vi "Parse Uplink.vi"(8 "error in (no error)":errorcluster, 10 "Uplink":u8[][](array[numeric]) format="%02x") -> (0 "error out":errorcluster, 1 "Data":string, 2 "Response Code":string, 3 "Response Token":string, 4 "tChecksum Valid":bool, 5 "CP_DATA":u8[](array[numeric]), 6 "bChecksum Valid":bool)   [LabVIEW 2020]
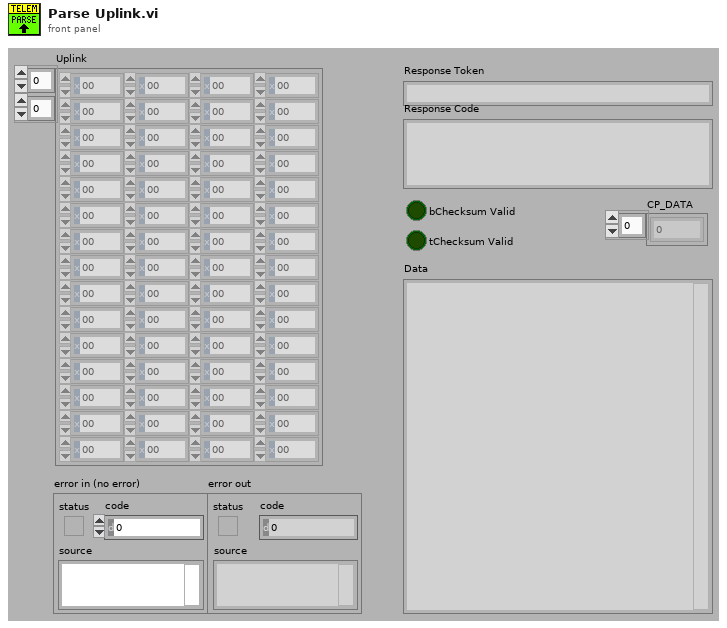
[diagram p1: front panel]
types:
  T1 = cluster{"FirstBlockFlag":u8, "respToken":u8, "cmdToken":u16, "cmdData":u8[], "b1ChkSum":u8, "tChkSum":u8, "tChkSumCalc":u8, "b1ChkSumCalc":u8}
  T2 = cluster{"Boolean array[0]":bool, "Boolean array[1]":bool, "Boolean array[2]":bool, "Boolean array[3]":bool, "Boolean array[4]":bool, "Boolean array[5]":bool, "Boolean array[6]":bool, "Boolean array[7]":bool}
  T3 = cluster{"Boolean array[0]":bool, "Boolean array[1]":bool, "Boolean array[2]":bool, "Boolean array[3]":bool, "Boolean array[4]":bool, "Boolean array[5]":bool, "Boolean array[6]":bool, "Boolean array[7]":bool, "Boolean array[8]":bool, "Boolean array[9]":bool, "Boolean array[10]":bool, "Boolean array[11]":bool, "Boolean array[12]":bool, "Boolean array[13]":bool, "Boolean array[14]":bool, "Boolean array[15]":bool}
  T4 = cluster{"DATA[0]":u8, "DATA[1]":u8, "DATA[2]":u8, "DATA[3]":u8, "DATA[4]":u8, "DATA[5]":u8, "DATA[6]":u8, "DATA[7]":u8}
  T5 = cluster{"[0]":string, "[1]":string, "[2]":string, "[3]":string, "[4]":string, "[5]":string, "[6]":string, "[7]":string, "[8]":string, "[9]":string}
  T6 = cluster{"DATA[0]":u8, "DATA[1]":u8, "DATA[2]":u8, "DATA[3]":u8, "DATA[4]":u8, "DATA[5]":u8, "DATA[6]":u8, "DATA[7]":u8, "DATA[8]":u8, "DATA[9]":u8, "DATA[10]":u8, "DATA[11]":u8, "DATA[12]":u8, "DATA[13]":u8, "DATA[14]":u8, "DATA[15]":u8}
  T7 = cluster{"[0]":u8, "[1]":u8, "[2]":u8, "[3]":u8, "[4]":u8, "[5]":u8, "[6]":u8, "[7]":u8, "[8]":u8, "[9]":u8, "[10]":u8, "[11]":u8, "[12]":u8, "[13]":u8, "[14]":u8, "[15]":u8, "[16]":u8, "[17]":u8, "[18]":u8, "[19]":u8, "[20]":u8, "[21]":u8, "[22]":u8, "[23]":u8, "[24]":u8, "[25]":u8, "[26]":u8, "[27]":u8, "[28]":u8, "[29]":u8, "[30]":u8, "[31]":u8, "[32]":u8, "[33]":u8, "[34]":u8, "[35]":u8, "[36]":u8, "[37]":u8, "[38]":u8, "[39]":u8, "[40]":u8, "[41]":u8, "[42]":u8, "[43]":u8, "[44]":u8, "[45]":u8, "[46]":u8, "[47]":u8, "[48]":u8, "[49]":u8, "[50]":u8, "[51]":u8, "[52]":u8, "[53]":u8}
  T8 = cluster{"DATA[0]":u8, "DATA[1]":u8, "DATA[2]":u8, "DATA[3]":u8, "DATA[4]":u8, "DATA[5]":u8, "DATA[6]":u8, "DATA[7]":u8, "DATA[8]":u8, "DATA[9]":u8, "DATA[10]":u8, "DATA[11]":u8, "DATA[12]":u8, "DATA[13]":u8, "DATA[14]":u8, "DATA[15]":u8, "DATA[16]":u8, "DATA[17]":u8, "DATA[18]":u8, "DATA[19]":u8, "DATA[20]":u8, "DATA[21]":u8, "DATA[22]":u8, "DATA[23]":u8, "DATA[24]":u8, "DATA[25]":u8, "DATA[26]":u8, "DATA[27]":u8, "DATA[28]":u8, "DATA[29]":u8, "DATA[30]":u8, "DATA[31]":u8, "DATA[32]":u8, "DATA[33]":u8, "DATA[34]":u8, "DATA[35]":u8, "DATA[36]":u8, "DATA[37]":u8, "DATA[38]":u8, "DATA[39]":u8, "DATA[40]":u8, "DATA[41]":u8, "DATA[42]":u8, "DATA[43]":u8, "DATA[44]":u8, "DATA[45]":u8, "DATA[46]":u8}
  T9 = cluster{"DATA[0]":u8, "DATA[1]":u8, "DATA[2]":u8, "DATA[3]":u8, "DATA[4]":u8, "DATA[5]":u8, "DATA[6]":u8, "DATA[7]":u8, "DATA[8]":u8, "DATA[9]":u8, "DATA[10]":u8, "DATA[11]":u8, "DATA[12]":u8, "DATA[13]":u8, "DATA[14]":u8, "DATA[15]":u8, "DATA[16]":u8, "DATA[17]":u8, "DATA[18]":u8, "DATA[19]":u8, "DATA[20]":u8, "DATA[21]":u8, "DATA[22]":u8, "DATA[23]":u8}
  T10 = cluster{"Boolean array[0]":bool, "Boolean array[1]":bool, "Boolean array[2]":bool, "Boolean array[3]":bool, "Boolean array[4]":bool, "Boolean array[5]":bool, "Boolean array[6]":bool, "Boolean array[7]":bool, "Boolean array[8]":bool}
  T11 = cluster{"[0]":u8, "[1]":u8, "[2]":u8, "[3]":u8, "[4]":u8, "[5]":u8, "[6]":u8, "[7]":u8, "[8]":u8, "[9]":u8}
  T12 = cluster{"DATA[0]":u8, "DATA[1]":u8, "DATA[2]":u8, "DATA[3]":u8, "DATA[4]":u8, "DATA[5]":u8, "DATA[6]":u8, "DATA[7]":u8, "DATA[8]":u8}
  T13 = cluster{"[0]":u8, "[1]":u8, "[2]":u8, "[3]":u8, "[4]":u8, "[5]":u8, "[6]":u8, "[7]":u8, "[8]":u8, "[9]":u8, "[10]":u8, "[11]":u8, "[12]":u8, "[13]":u8, "[14]":u8, "[15]":u8, "[16]":u8, "[17]":u8, "[18]":u8, "[19]":u8, "[20]":u8, "[21]":u8, "[22]":u8, "[23]":u8, "[24]":u8, "[25]":u8, "[26]":u8, "[27]":u8, "[28]":u8, "[29]":u8, "[30]":u8, "[31]":u8, "[32]":u8, "[33]":u8, "[34]":u8, "[35]":u8, "[36]":u8, "[37]":u8}
  T14 = cluster{"[0]":u8, "[1]":u8, "[2]":u8, "[3]":u8, "[4]":u8, "[5]":u8}
  T15 = cluster{"DATA[0]":u8, "DATA[1]":u8, "DATA[2]":u8, "DATA[3]":u8, "DATA[4]":u8, "DATA[5]":u8}
  T16 = cluster{"DATA[0]":u8, "DATA[1]":u8, "DATA[2]":u8, "DATA[3]":u8, "DATA[4]":u8, "DATA[5]":u8, "DATA[6]":u8, "DATA[7]":u8, "DATA[8]":u8, "DATA[9]":u8, "DATA[10]":u8, "DATA[11]":u8, "DATA[12]":u8, "DATA[13]":u8, "DATA[14]":u8, "DATA[15]":u8, "DATA[16]":u8}
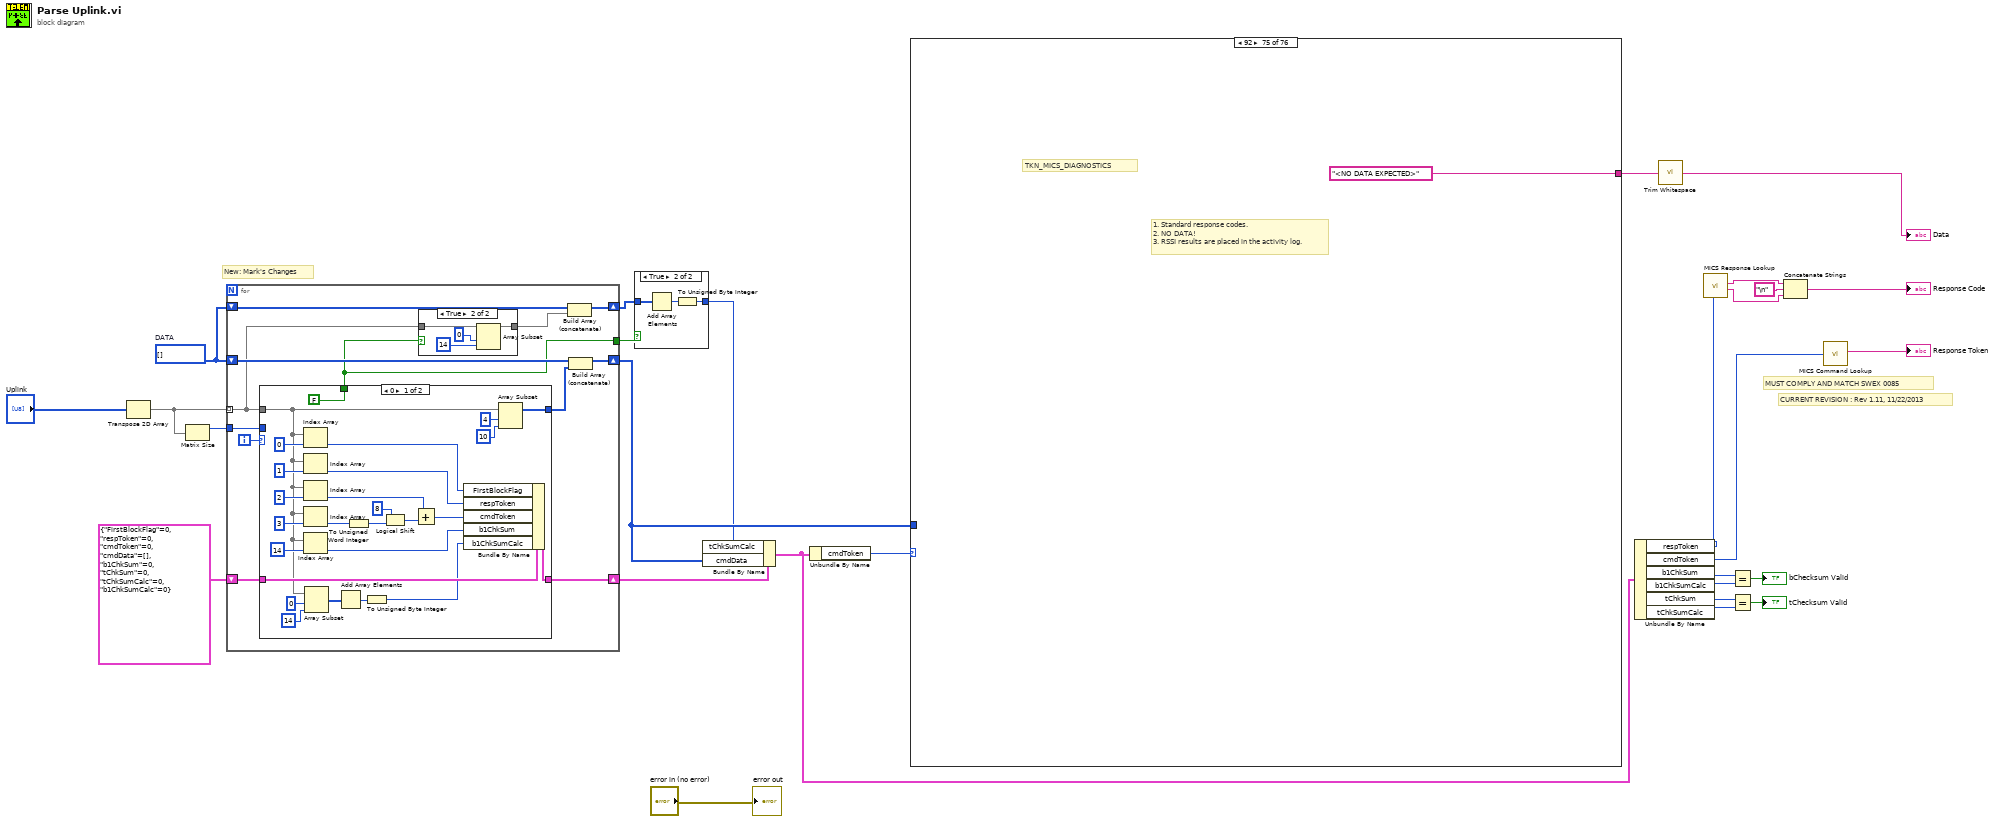
[diagram p0: block diagram]
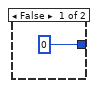
[diagram p2: hidden frame]
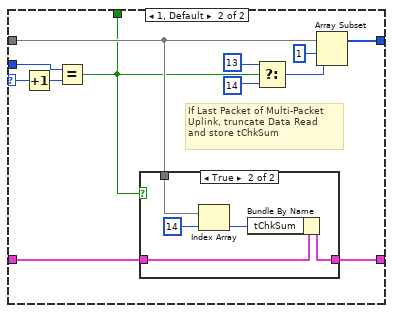
[diagram p4: hidden frame]
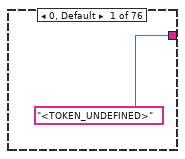
[diagram p6: hidden frame]
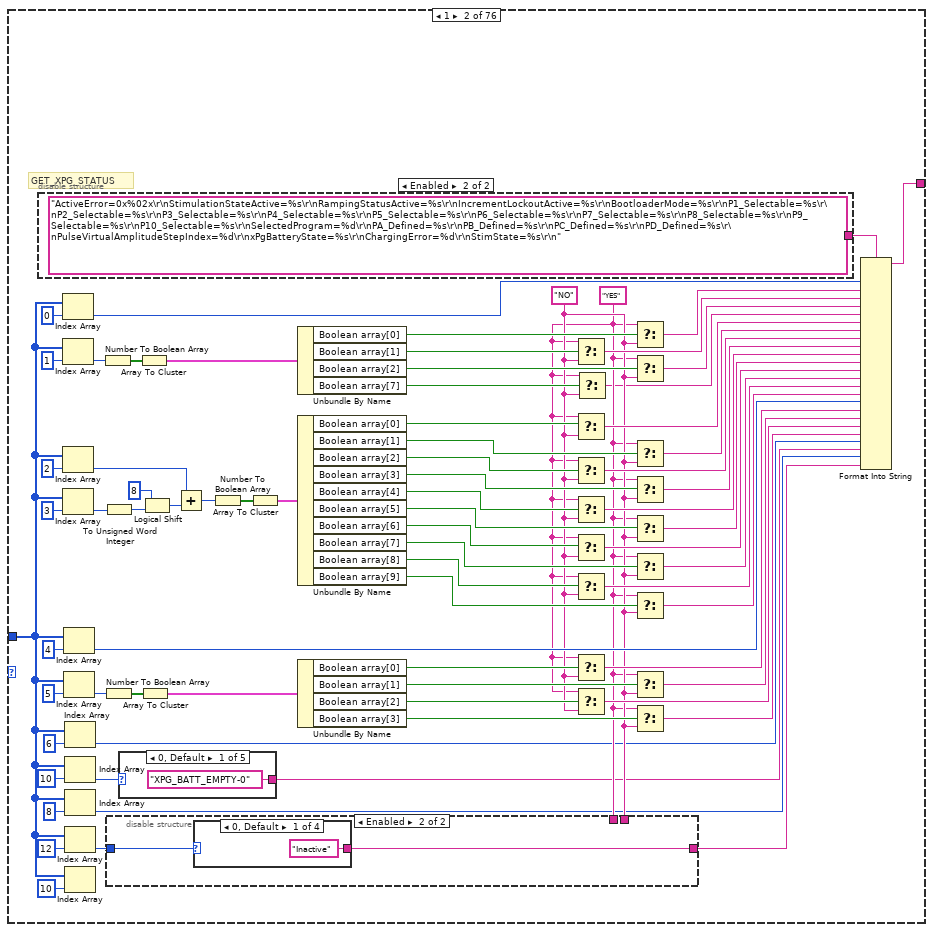
[diagram p7: hidden frame]
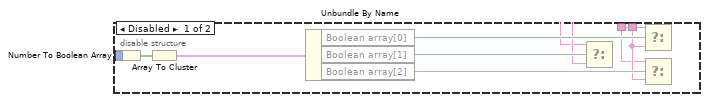
[diagram p8: hidden frame]
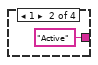
[diagram p9: hidden frame]
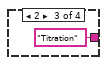
[diagram p10: hidden frame]
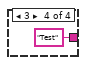
[diagram p11: hidden frame]
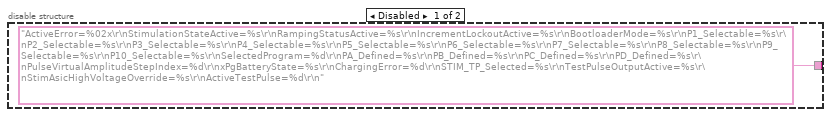
[diagram p12: hidden frame]
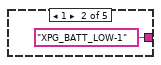
[diagram p13: hidden frame]
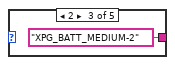
[diagram p14: hidden frame]
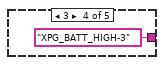
[diagram p15: hidden frame]
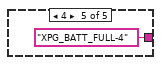
[diagram p16: hidden frame]
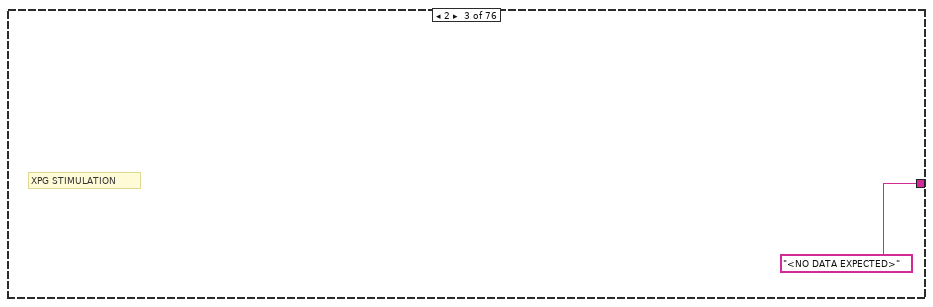
[diagram p17: hidden frame]
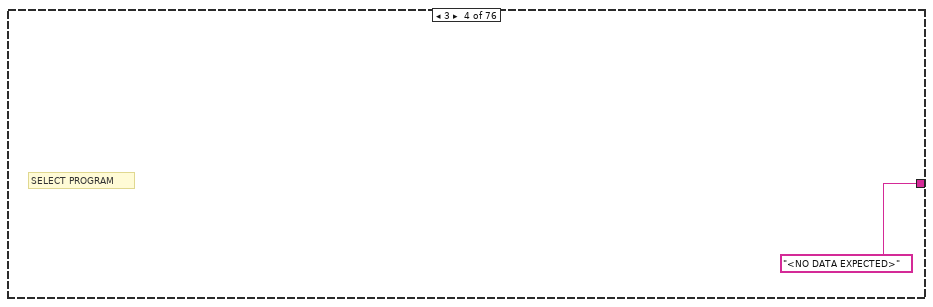
[diagram p18: hidden frame]
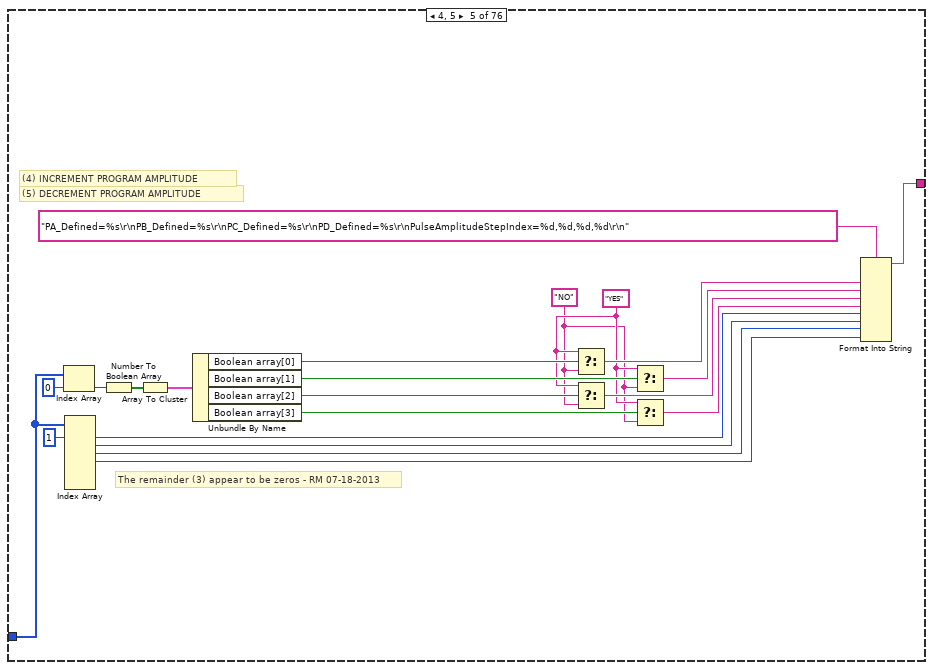
[diagram p19: hidden frame]
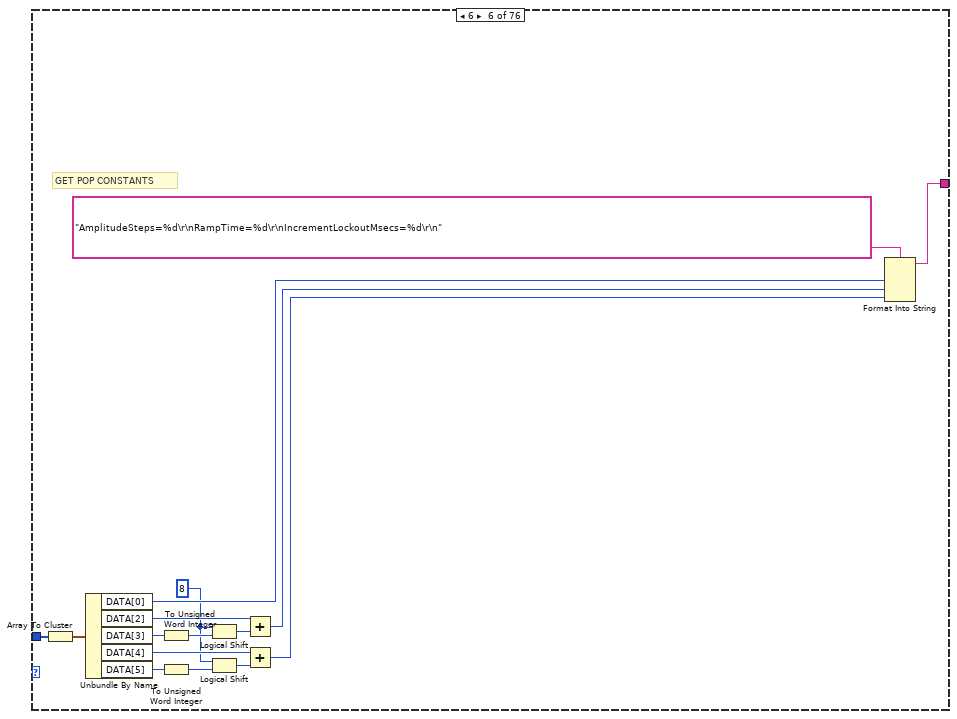
[diagram p20: hidden frame]
diagram:
  w12 = u8[] []  # DATA
  # "CURRENT REVISION : Rev 1.11, 11/22/2013"
  # "MUST COMPLY AND MATCH SWEX 0085"
  # "New: Mark's Changes"
  n1 = Transpose 2D Array(2D array="Uplink") -> (transposed array=w11:u8[][])
  n2 = Matrix Size(0:w11) -> (1:w9:i32)  [unwired: 1 out]
  n3 = for {
    tunnel: w11 -> [w31] mode=indexing
    shift-right: [w35] -> w28
    shift-left: w12 -> [w36]
    shift-right: [w38] -> w10
    shift-left: T1 {"FirstBlockFlag"=0, "respToken"=0, "cmdToken"=0, "cmdData"=[], "b1ChkSum"=0, "tChkSum"=0, "tChkSumCalc"=0, "b1ChkSumCalc"=0} -> [w39]
    tunnel: w9 -> [w37]
    shift-right: [w32] -> w13
    shift-left: w12 -> [w33]
    tunnel: [w29] -> w14
    i -> [w40]
    n4 = case shown="0" w40 {
      selector: w40 -> [_ w83]
      tunnel: w31 -> [w49 w73]
      tunnel: [w69 w79] -> w34
      tunnel: w39 -> [w63 w74]
      tunnel: [w62 w75] -> w38
      tunnel: w37 -> [_ w81]
      tunnel: [FALSE w72] -> w29
      frame 0 {
        n5 = Index Array(array=w49, index=0) -> (element=w61:u8)
        n6 = Index Array(array=w49, index=1) -> (element=w58:u8)
        n7 = Index Array(array=w49, index=2) -> (element=w53:u8)
        n8 = Index Array(array=w49, index=3) -> (element=w57:u8)
        n9 = Index Array(array=w49, index=14) -> (element=w60:u8)
        n10 = Array Subset(array=w49, index=0, length=14) -> (w46:u8[])
        n11 = Add Array Elements(numeric array=w46) -> (sum=w48:u8)
        n12 = To Unsigned Word Integer(number=w57) -> (unsigned 16bit integer=w59:u16)
        n13 = To Unsigned Byte Integer(number=w48) -> (unsigned 8bit integer=w47:u8)
        n14 = Logical Shift(y=i8 8, x=w59) -> (x << y=w55:u16)
        n15 = Add(x=w53, y=w55) -> (x+y=w54:u16)
        n16 = Bundle By Name(cluster=w63, "FirstBlockFlag"=w61, "respToken"=w58, "cmdToken"=w54, "b1ChkSum"=w60, "b1ChkSumCalc"=w47) -> (w62:T1)
        n17 = Array Subset(array=w49, index=4, length=10) -> (w69:u8[])
      }
      frame 1, Default {
        # "If Last Packet of Multi-Packet\nUplink, truncate Data Read\nand store tChkSum"
        n18 = Increment(x=w83) -> (x+1=w82:i32)
        n19 = Equal?(x=w81, y=w82) -> (x = y?=w72:bool)
        n20 = case shown="True" w72 {
          tunnel: [w84 w88] -> w75
          tunnel: w74 -> [w84 w89]
          tunnel: w73 -> [_ w86]
          frame False {
          }
          frame True {
            n21 = Index Array(array=w86, index=14) -> (element=w87:u8)
            n22 = Bundle By Name(cluster=w89, "tChkSum"=w87) -> (w88:T1)
          }
        }
        n23 = Select(t=13 ("length"), s=w72, f=14 ("length")) -> (s? t:f=w78:i32)
        n24 = Array Subset(array=w73, index=1, length=w78) -> (w79:u8[])
      }
    }
    n25 = case shown="True" w29 {
      tunnel: w31 -> [w41 w44]
      tunnel: [w41 w43] -> w30
      frame False {
      }
      frame True {
        n26 = Array Subset(array=w44, index=0, length=14) -> (w43:u8[])
      }
    }
    n27 = Build Array (concatenate)(w33, w30) -> (w32:u8[])
    n28 = Build Array (concatenate)(w36, w34) -> (w35:u8[])
  }
  n29 = case shown="True" w14 {
    tunnel: w13 -> [_ w91]
    tunnel: [u16 0 ("CRC16r") w92] -> w15
    frame False {
    }
    frame True {
      n30 = Add Array Elements(numeric array=w91) -> (sum=w93:u8)
      n31 = To Unsigned Byte Integer(number=w93) -> (unsigned 8bit integer=w92:u8)
    }
  }
  n32 = Bundle By Name(cluster=w10, "tChkSumCalc"=w15, "cmdData"=w28) -> (w19:T1)
  n33 = Unbundle By Name(w19) -> ("cmdToken"=w16:u16)
  n34 = case shown="92" w16 {
    tunnel: w28 -> [_ w104 _ _ w203 w221 w230 w312 w358 w363 w368 w384 _ w403 w408 w413 _ w419 w424 _ w439 w465 _ _ w473 _ w610 _ w635 _ w785 _ w794 _ w852 _ w899 _ w925 _ _ w954 w988 w1010 _ w1018 _ w1028 w1033 w1054 _ w1144 _ w1192 _ w1197 _ w1257 _ w1313 _ w1318 _ _ _ w1336 _ _ _ _ w1353 _ w1409 w1417 _ _]
    tunnel: ["<TOKEN_UNDEFINED>" w166 "<NO DATA EXPECTED>" "<NO DATA EXPECTED>" w213 w228 w289 w345 w359 w364 w369 w398 "<NO DATA EXPECTED>" w404 w409 w414 "<NO DATA EXPECTED>" w420 w425 "<NO DATA EXPECTED>" w440 w452 "<NO DATA EXPECTED>" "<NO DATA EXPECTED>" w512 "<NO DATA EXPECTED>" w613 "<NO DATA EXPECTED>" w700 "<NO DATA EXPECTED>" w789 "<NO DATA EXPECTED>" w799 "<NO DATA EXPECTED>" w857 "<NO DATA EXPECTED>" w902 "<NO DATA EXPECTED>" w928 "<NO DATA EXPECTED>" "<NO DATA EXPECTED>" ("format string") w955 w990 w1012 "<NO DATA EXPECTED>" w1022 "<NO DATA EXPECTED>" w1030 w1037 w1085 "<NO DATA EXPECTED>" w1145 "<NO DATA EXPECTED>" w1193 "<NO DATA EXPECTED>" w1205 "<NO DATA EXPECTED>" w1264 "<NO DATA EXPECTED>" w1314 "<NO DATA EXPECTED>" w1326 _ _ "<NO DATA EXPECTED>" w1344 _ _ _ _ w1354 "<NO DATA EXPECTED>" w1411 w1423 "<NO DATA EXPECTED>" "<TOKEN_UNDEFINED (0x7FAA)>"] -> w27
    frame 0, Default {
    }
    frame 1 {
      w102 = "NO"
      w101 = "YES"
      # "GET_XPG_STATUS"
      n35 = disable-structure shown="Enabled" {
        disable-tunnel: ["ActiveError=%02x\r\nStimulationStateActive=%s\r\nRampingStatusActive=%s\r\nIncrementLockoutActive=%s\r\nBootloaderMode=%s\r\nP1_Selectable=%s\r\nP2_Selectable=%s\r\nP3_Selectable=%s\r\nP4_Selectable=%s\r\nP5_Selectable=%s\r\nP6_Selectable=%s\r\nP7_Selectable=%s\r\nP8_Selectable=%s\r\nP9_Selectable=%s\r\nP10_Selectable=%s\r\nSelectedProgram=%d\r\nPA_Defined=%s\r\nPB_Defined=%s\r\nPC_Defined=%s\r\nPD_Defined=%s\r\nPulseVirtualAmplitudeStepIndex=%d\r\nxPgBatteryState=%s\r\nChargingError=%d\r\nSTIM_TP_Selected=%s\r\nTestPulseOutputActive=%s\r\nStimAsicHighVoltageOverride=%s\r\nActiveTestPulse=%d\r\n" ("format string") "ActiveError=0x%02x\r\nStimulationStateActive=%s\r\nRampingStatusActive=%s\r\nIncrementLockoutActive=%s\r\nBootloaderMode=%s\r\nP1_Selectable=%s\r\nP2_Selectable=%s\r\nP3_Selectable=%s\r\nP4_Selectable=%s\r\nP5_Selectable=%s\r\nP6_Selectable=%s\r\nP7_Selectable=%s\r\nP8_Selectable=%s\r\nP9_Selectable=%s\r\nP10_Selectable=%s\r\nSelectedProgram=%d\r\nPA_Defined=%s\r\nPB_Defined=%s\r\nPC_Defined=%s\r\nPD_Defined=%s\r\nPulseVirtualAmplitudeStepIndex=%d\r\nxPgBatteryState=%s\r\nChargingError=%d\r\nStimState=%s\r\n" ("format string")] -> w95
        frame Disabled {
        }
        frame Enabled {
        }
      }
      n36 = Index Array(array=w104, index=0) -> (element=w167:u8)
      n37 = Index Array(array=w104, index=1) -> (element=w151:u8)
      n38 = Index Array(array=w104, index=2) -> (element=w139:u8)
      n39 = Index Array(array=w104, index=3) -> (element=w140:u8)
      n40 = Index Array(array=w104, index=4) -> (element=w124:u8)
      n41 = Index Array(array=w104, index=5) -> (element=w122:u8)
      n42 = Index Array(array=w104, index=6) -> (element=w99:u8)
      n43 = Index Array(array=w104, index=10) -> (element=w109:u8)
      n44 = Index Array(array=w104, index=8) -> (element=w97:u8)
      n45 = Index Array(array=w104, index=12) -> (element=w106:u8)
      n46 = Index Array(array=w104, index=10) -> ()  [unwired: 1 out]
      n47 = Number To Boolean Array(number=w151) -> (Boolean array=w150:bool[])
      n48 = To Unsigned Word Integer(number=w140) -> (unsigned 16bit integer=w143:u16)
      n49 = Number To Boolean Array(number=w122) -> (Boolean array=w121:bool[])
      n50 = disable-structure shown="Enabled" {
        disable-tunnel: w106 -> [w176 w178]
        disable-tunnel: w102 -> [w170 _]
        disable-tunnel: w101 -> [w169 _]
        disable-tunnel: [_ w177] -> w96
        frame Disabled {
          n51 = Number To Boolean Array(number=w176) -> (Boolean array=w175:bool[])
          n52 = Array To Cluster(array=w175) -> (cluster=w174:T2)
          n53 = Unbundle By Name(w174) -> ("Boolean array[0]"=w173:bool, "Boolean array[1]"=w172:bool, "Boolean array[2]"=w171:bool)
          n54 = Select(t=w169, s=w172, f=w170) -> ()  [unwired: 1 out]
          n55 = Select(t=w169, s=w173, f=w170) -> ()  [unwired: 1 out]
          n56 = Select(t=w169, s=w171, f=w170) -> ()  [unwired: 1 out]
        }
        frame Enabled {
          n57 = case shown="0, Default" w178 {
            tunnel: ["Inactive" "Active" "Titration" "Test"] -> w177
            frame 0, Default {
            }
            frame 1 {
            }
            frame 2 {
            }
            frame 3 {
            }
          }
        }
      }
      n58 = case shown="0, Default" w109 {
        tunnel: ["XPG_BATT_EMPTY-0" "XPG_BATT_LOW-1" "XPG_BATT_MEDIUM-2" "XPG_BATT_HIGH-3" "XPG_BATT_FULL-4"] -> w98
        frame 0, Default {
        }
        frame 1 {
        }
        frame 2 {
        }
        frame 3 {
        }
        frame 4 {
        }
      }
      n59 = Array To Cluster(array=w150) -> (cluster=w149:T2)
      n60 = Array To Cluster(array=w121) -> (cluster=w120:T2)
      n61 = Logical Shift(y=i8 8, x=w143) -> (x << y=w141:u16)
      n62 = Add(x=w139, y=w141) -> (x+y=w137:u16)
      n63 = Number To Boolean Array(number=w137) -> (Boolean array=w138:bool[])
      n64 = Array To Cluster(array=w138) -> (cluster=w136:T3)
      n65 = Unbundle By Name(w149) -> ("Boolean array[0]"=w148:bool, "Boolean array[1]"=w147:bool, "Boolean array[2]"=w146:bool, "Boolean array[7]"=w103:bool)
      n66 = Unbundle By Name(w136) -> ("Boolean array[0]"=w135:bool, "Boolean array[1]"=w134:bool, "Boolean array[2]"=w133:bool, "Boolean array[3]"=w132:bool, "Boolean array[4]"=w131:bool, "Boolean array[5]"=w130:bool, "Boolean array[6]"=w129:bool, "Boolean array[7]"=w128:bool, "Boolean array[8]"=w127:bool, "Boolean array[9]"=w126:bool)
      n67 = Unbundle By Name(w120) -> ("Boolean array[0]"=w119:bool, "Boolean array[1]"=w118:bool, "Boolean array[2]"=w117:bool, "Boolean array[3]"=w116:bool)
      n68 = Select(t=w101, s=w147, f=w102) -> (s? t:f=w164:string)
      n69 = Select(t=w101, s=w135, f=w102) -> (s? t:f=w162:string)
      n70 = Select(t=w101, s=w133, f=w102) -> (s? t:f=w160:string)
      n71 = Select(t=w101, s=w131, f=w102) -> (s? t:f=w158:string)
      n72 = Select(t=w101, s=w129, f=w102) -> (s? t:f=w156:string)
      n73 = Select(t=w101, s=w127, f=w102) -> (s? t:f=w154:string)
      n74 = Select(t=w101, s=w119, f=w102) -> (s? t:f=w115:string)
      n75 = Select(t=w101, s=w117, f=w102) -> (s? t:f=w113:string)
      n76 = Select(t=w101, s=w103, f=w102) -> (s? t:f=w100:string)
      n77 = Select(t=w101, s=w148, f=w102) -> (s? t:f=w165:string)
      n78 = Select(t=w101, s=w146, f=w102) -> (s? t:f=w163:string)
      n79 = Select(t=w101, s=w134, f=w102) -> (s? t:f=w161:string)
      n80 = Select(t=w101, s=w132, f=w102) -> (s? t:f=w159:string)
      n81 = Select(t=w101, s=w130, f=w102) -> (s? t:f=w157:string)
      n82 = Select(t=w101, s=w128, f=w102) -> (s? t:f=w155:string)
      n83 = Select(t=w101, s=w126, f=w102) -> (s? t:f=w153:string)
      n84 = Select(t=w101, s=w118, f=w102) -> (s? t:f=w114:string)
      n85 = Select(t=w101, s=w116, f=w102) -> (s? t:f=w112:string)
      n86 = Format Into String(format string=w95, w167, w165, w164, w163, w100, w162, w161, w160, w159, w158, w157, w156, w155, w154, w153, w124, w115, w114, w113, w112, w99, w98, w97, w96) -> (resulting string=w166:string)  [unwired: 2 in, 1 out]
    }
    frame 2 {
      # "XPG STIMULATION"
    }
    frame 3 {
      # "SELECT PROGRAM"
    }
    frame 4, 5 {
      w196 = "NO"
      w197 = "YES"
      # "(5) DECREMENT PROGRAM AMPLITUDE"
      # "(4) INCREMENT PROGRAM AMPLITUDE"
      # "The remainder (3) appear to be zeros - RM 07-18-2013"
      n87 = Index Array(array=w203, index=0) -> (element=w211:u8)
      n88 = Index Array(array=w203, index #1=1 ("index")) -> (element #1=w198:u8, element #2=w194:u8, element #3=w193:u8, element #4=w192:u8)  [unwired: 6 in, 3 out]
      n89 = Number To Boolean Array(number=w211) -> (Boolean array=w210:bool[])
      n90 = Array To Cluster(array=w210) -> (cluster=w209:T2)
      n91 = Unbundle By Name(w209) -> ("Boolean array[0]"=w208:bool, "Boolean array[1]"=w207:bool, "Boolean array[2]"=w206:bool, "Boolean array[3]"=w205:bool)
      n92 = Select(t=w197, s=w208, f=w196) -> (s? t:f=w202:string)
      n93 = Select(t=w197, s=w206, f=w196) -> (s? t:f=w200:string)
      n94 = Select(t=w197, s=w207, f=w196) -> (s? t:f=w201:string)
      n95 = Select(t=w197, s=w205, f=w196) -> (s? t:f=w199:string)
      n96 = Format Into String(format string="PA_Defined=%s\r\nPB_Defined=%s\r\nPC_Defined=%s\r\nPD_Defined=%s\r\nPulseAmplitudeStepIndex=%d,%d,%d,%d\r\n", w202, w201, w200, w199, w198, w194, w193, w192) -> (resulting string=w213:string)  [unwired: 2 in, 1 out]
    }
    frame 6 {
      w214 = i8 8 ("y")
      # "GET POP CONSTANTS"
      n97 = Array To Cluster(array=w221) -> (cluster=w220:T4)
      n98 = Unbundle By Name(w220) -> ("DATA[0]"=w219:u8, "DATA[2]"=w218:u8, "DATA[3]"=w217:u8, "DATA[4]"=w216:u8, "DATA[5]"=w215:u8)
      n99 = To Unsigned Word Integer(number=w217) -> (unsigned 16bit integer=w227:u16)
      n100 = To Unsigned Word Integer(number=w215) -> (unsigned 16bit integer=w225:u16)
      n101 = Logical Shift(y=w214, x=w227) -> (x << y=w226:u16)
      n102 = Logical Shift(y=w214, x=w225) -> (x << y=w224:u16)
      n103 = Add(x=w218, y=w226) -> (x+y=w223:u16)
      n104 = Add(x=w216, y=w224) -> (x+y=w222:u16)
      n105 = Format Into String(format string="AmplitudeSteps=%d\r\nRampTime=%d\r\nIncrementLockoutMsecs=%d\r\n", w219, w223, w222) -> (resulting string=w228:string)  [unwired: 2 in, 1 out]
    }
    frame 7 {
      w232 = "NO"
      w270 = "YES"
      # "Convert MS DateTime\nto LV DateTime"
      # "GET PPC CONSTANTS"
      n106 = Array Subset(array=w230, index=0, length=30) -> (w286:u8[])
      n107 = Index Array(array=w230, index=30) -> (element=w278:u8)
      n108 = Index Array(array=w230, index=31) -> (element=w279:u8)
      n109 = Index Array(array=w230, index=32) -> (element=w275:u8)
      n110 = Index Array(array=w230, index=33) -> (element=w273:u8)
      n111 = Index Array(array=w230, index=34) -> (element=w257:u8)
      n112 = Index Array(array=w230, index=35) -> (element=w258:u8)
      n113 = Index Array(array=w230, index=36) -> (element=w249:u8)
      n114 = Index Array(array=w230, index=37) -> (element=w250:u8)
      n115 = Array Subset(array=w230, index=38, length=8) -> (w245:u8[])
      n116 = Index Array(array=w230, index=46) -> (element=w235:u8)
      n117 = Number To Boolean Array(number=w273) -> (Boolean array=w272:bool[])
      n118 = To Unsigned Word Integer(number=w279) -> (unsigned 16bit integer=w282:u16)
      n119 = To Unsigned Word Integer(number=w258) -> (unsigned 16bit integer=w261:u16)
      n120 = To Unsigned Word Integer(number=w250) -> (unsigned 16bit integer=w253:u16)
      n121 = Byte Array To String(unsigned byte array=w286) -> (string=w285:string)
      n122 = Array To Cluster(array=w272) -> (cluster=w271:T2)
      n123 = Logical Shift(y=i8 8, x=w282) -> (x << y=w280:u16)
      n124 = Logical Shift(y=i8 8, x=w261) -> (x << y=w259:u16)
      n125 = Logical Shift(y=i8 8, x=w253) -> (x << y=w251:u16)
      n126 = for {
        tunnel: w245 -> [w298] mode=indexing
        shift-right: [w292] -> w240
        shift-left: u64 0 ("y") -> [w293]
        tunnel: i8 8 ("y") -> [w296]
        i -> [w297]
        n127 = To Unsigned Quad Integer(1:w298) -> (0:w291:u64)
        n128 = Multiply(x=w296, y=w297) -> (x*y=w295:i32)
        n129 = Logical Shift(y=w295, x=w291) -> (x << y=w294:u64)
        n130 = Add(x=w293, y=w294) -> (x+y=w292:u64)
      }
      n131 = Add(x=w278, y=w280) -> (x+y=w277:u16)
      n132 = Unbundle By Name(w271) -> ("Boolean array[0]"=w268:bool, "Boolean array[1]"=w269:bool, "Boolean array[2]"=w267:bool)
      n133 = Add(x=w257, y=w259) -> (x+y=w256:u16)
      n134 = Add(x=w249, y=w251) -> (x+y=w248:u16)
      n135 = Select(t=w270, s=w268, f=w232) -> (s? t:f=w266:string)
      n136 = Select(t=w270, s=w267, f=w232) -> (s? t:f=w264:string)
      n137 = Multiply(x=u64 1904 ("y"), y=u64 31556926) -> (x*y=w238:u64)
      n138 = Quotient & Remainder(x=w240, y=u64 10000000) -> (floor(x/y)=w231:u64)  [unwired: 1 out]
      n139 = Select(t=w270, s=w269, f=w232) -> (s? t:f=w265:string)
      n140 = Subtract(x=w231, y=w238) -> (x-y=w234:u64)
      n141 = Format Date/Time String(seconds (now)=w234, UTC format=FALSE) -> (date/time string=w233:string)  [unwired: 1 in]
      n142 = Format Into String(format string="PPCText=%s\r\nPulseWidthStep=%d\r\nAmplitudeSteps=%d\r\nAllowIndividualPulseAmplitudeModification=%s\r\nAllowIndividualPulseWidthModification=%s\r\nAllowProgramFrequencyModification=%s\r\nRampTime=%d\r\nIncrementalLockoutMsecs=%d\r\nImplantDateTime=%s\r\nReplacementIntervalMonths=%d\r\n", w285, w277, w275, w266, w265, w264, w256, w248, w233, w235) -> (resulting string=w289:string)  [unwired: 2 in, 1 out]
    }
    frame 8 {
      w324 = "NO"
      w323 = "YES"
      # "GET_PROGRAM_NAMES"
      n143 = Index Array(array=w312, index=0) -> (element=w338:u8)
      n144 = Index Array(array=w312, index=1) -> (element=w339:u8)
      n145 = To Unsigned Word Integer(number=w339) -> (unsigned 16bit integer=w342:u16)
      n146 = Logical Shift(y=i8 8, x=w342) -> (x << y=w340:u16)
      n147 = Add(x=w338, y=w340) -> (x+y=w336:u16)
      n148 = for {
        N: 10 -> [_]
        tunnel: w312 -> [w355]
        tunnel: [w347] -> w311 mode=indexing
        i -> [w353]
        n149 = Multiply(x=16, y=w353) -> (x*y=w351:i32)
        n150 = Add(x=2, y=w351) -> (x+y=w349:i32)
        n151 = Array Subset(array=w355, index=w349, length=10) -> (w348:u8[])
        n152 = Byte Array To String(unsigned byte array=w348) -> (string=w347:string)
      }
      n153 = Number To Boolean Array(number=w336) -> (Boolean array=w337:bool[])
      n154 = Array To Cluster(array=w337) -> (cluster=w335:T3)
      n155 = Unbundle By Name(w335) -> ("Boolean array[0]"=w334:bool, "Boolean array[1]"=w333:bool, "Boolean array[2]"=w332:bool, "Boolean array[3]"=w331:bool, "Boolean array[4]"=w330:bool, "Boolean array[5]"=w329:bool, "Boolean array[6]"=w328:bool, "Boolean array[7]"=w327:bool, "Boolean array[8]"=w326:bool, "Boolean array[9]"=w325:bool)
      n156 = Array To Cluster(array=w311) -> (cluster=w310:T5)
      n157 = Unbundle(w310) -> ("[0]"=w308:string, "[1]"=w307:string, "[2]"=w306:string, "[3]"=w305:string, "[4]"=w304:string, "[5]"=w303:string, "[6]"=w302:string, "[7]"=w301:string, "[8]"=w300:string, "[9]"=w299:string)
      n158 = Select(t=w323, s=w334, f=w324) -> (s? t:f=w322:string)
      n159 = Select(t=w323, s=w332, f=w324) -> (s? t:f=w320:string)
      n160 = Select(t=w323, s=w330, f=w324) -> (s? t:f=w318:string)
      n161 = Select(t=w323, s=w328, f=w324) -> (s? t:f=w316:string)
      n162 = Select(t=w323, s=w326, f=w324) -> (s? t:f=w314:string)
      n163 = Select(t=w323, s=w333, f=w324) -> (s? t:f=w321:string)
      n164 = Select(t=w323, s=w331, f=w324) -> (s? t:f=w319:string)
      n165 = Select(t=w323, s=w329, f=w324) -> (s? t:f=w317:string)
      n166 = Select(t=w323, s=w327, f=w324) -> (s? t:f=w315:string)
      n167 = Select(t=w323, s=w325, f=w324) -> (s? t:f=w313:string)
      n168 = Format Into String(format string="P1_Selectable=%s\r\nP2_Selectable=%s\r\nP3_Selectable=%s\r\nP4_Selectable=%s\r\nP5_Selectable=%s\r\nP6_Selectable=%s\r\nP7_Selectable=%s\r\nP8_Selectable=%s\r\nP9_Selectable=%s\r\nP10_Selectable=%s\r\nP1_Name=%s\r\nP2_Name=%s\r\nP3_Name=%s\r\nP4_Name=%s\r\nP5_Name=%s\r\nP6_Name=%s\r\nP7_Name=%s\r\nP8_Name=%s\r\nP9_Name=%s\r\nP10_Name=%s\r\n", w322, w321, w320, w319, w318, w317, w316, w315, w314, w313, w308, w307, w306, w305, w304, w303, w302, w301, w300, w299) -> (resulting string=w345:string)  [unwired: 2 in, 1 out]
    }
    frame 9 {
      # "SET_PULSE_AMPLITUDE"
      n169 = Array To Cluster(array=w358) -> (cluster=w357:T4)
      n170 = Unbundle By Name(w357) -> ("DATA[0]"=w356:u8)
      n171 = Format Into String(format string="PulseAmplitudeStepIndex=%d\r\n", w356) -> (resulting string=w359:string)  [unwired: 2 in, 1 out]
    }
    frame 10 {
      # "INCREMENT_PULSE_AMPLITUDE"
      n172 = Array To Cluster(array=w363) -> (cluster=w362:T4)
      n173 = Unbundle By Name(w362) -> ("DATA[0]"=w361:u8)
      n174 = Format Into String(format string="PulseVirtualAmplitudeStepIndex=%d\r\n", w361) -> (resulting string=w364:string)  [unwired: 2 in, 1 out]
    }
    frame 11 {
      # "DECREMENT_PULSE_AMPLITUDE"
      n175 = Array To Cluster(array=w368) -> (cluster=w367:T4)
      n176 = Unbundle By Name(w367) -> ("DATA[0]"=w366:u8)
      n177 = Format Into String(format string="PulseVirtualAmplitudeStepIndex=%d\r\n", w366) -> (resulting string=w369:string)  [unwired: 2 in, 1 out]
    }
    frame 12 {
      w386 = "NO"
      w387 = "YES"
      # "GET_PULSE_WIDTHS"
      n178 = Array To Cluster(array=w384) -> (cluster=w385:T6)
      n179 = Unbundle By Name(w385) -> ("DATA[0]"=w383:u8, "DATA[3]"=w372:u8, "DATA[2]"=w371:u8, "DATA[5]"=w374:u8, "DATA[4]"=w373:u8, "DATA[7]"=w376:u8, "DATA[6]"=w375:u8, "DATA[9]"=w378:u8, "DATA[8]"=w377:u8)
      n180 = Join Numbers(hi=w372, lo=w371) -> ((hi.lo)=w382:u16)
      n181 = Join Numbers(hi=w374, lo=w373) -> ((hi.lo)=w381:u16)
      n182 = Join Numbers(hi=w376, lo=w375) -> ((hi.lo)=w380:u16)
      n183 = Join Numbers(hi=w378, lo=w377) -> ((hi.lo)=w379:u16)
      n184 = Number To Boolean Array(number=w383) -> (Boolean array=w397:bool[])
      n185 = Array To Cluster(array=w397) -> (cluster=w396:T2)
      n186 = Unbundle By Name(w396) -> ("Boolean array[0]"=w395:bool, "Boolean array[1]"=w394:bool, "Boolean array[2]"=w393:bool, "Boolean array[3]"=w392:bool)
      n187 = Select(t=w387, s=w395, f=w386) -> (s? t:f=w391:string)
      n188 = Select(t=w387, s=w393, f=w386) -> (s? t:f=w389:string)
      n189 = Select(t=w387, s=w394, f=w386) -> (s? t:f=w390:string)
      n190 = Select(t=w387, s=w392, f=w386) -> (s? t:f=w388:string)
      n191 = Format Into String(format string="PA_Defined=%s\r\nPB_Defined=%s\r\nPC_Defined=%s\r\nPD_Defined=%s\r\nPA_PulseWidth=%d\r\nPB_PulseWidth=%d\r\nPC_PulseWidth=%d\r\nPD_PulseWidth=%d\r\n", w391, w390, w389, w388, w382, w381, w380, w379) -> (resulting string=w398:string)  [unwired: 2 in, 1 out]
    }
    frame 13 {
      # "SET_PULSE_WIDTHS"
    }
    frame 14 {
      # "INCREMENT_PULSE_WIDTH"
      n192 = Array To Cluster(array=w403) -> (cluster=w402:T4)
      n193 = Unbundle By Name(w402) -> ("DATA[0]"=w401:u8)
      n194 = Format Into String(format string="PulseWidth=%d\r\n", w401) -> (resulting string=w404:string)  [unwired: 2 in, 1 out]
    }
    frame 15 {
      # "DECREMENT_PULSE_WIDTH"
      n195 = Array To Cluster(array=w408) -> (cluster=w407:T4)
      n196 = Unbundle By Name(w407) -> ("DATA[0]"=w406:u8)
      n197 = Format Into String(format string="PulseWidth=%d\r\n", w406) -> (resulting string=w409:string)  [unwired: 2 in, 1 out]
    }
    frame 16 {
      # "GET_PROGRAM_FREQUENCY"
      n198 = Array To Cluster(array=w413) -> (cluster=w412:T4)
      n199 = Unbundle By Name(w412) -> ("DATA[0]"=w411:u8)
      n200 = Format Into String(format string="ProgramFrequencyIndex=%d\r\n", w411) -> (resulting string=w414:string)  [unwired: 2 in, 1 out]
    }
    frame 17 {
      # "SET_PROGRAM_FREQUENCY"
    }
    frame 18 {
      # "INCREMENT_PROGRAM_FREQUENCY"
      n201 = Array To Cluster(array=w419) -> (cluster=w418:T4)
      n202 = Unbundle By Name(w418) -> ("DATA[0]"=w417:u8)
      n203 = Format Into String(format string="ProgramFrequencyIndex=%d\r\n", w417) -> (resulting string=w420:string)  [unwired: 2 in, 1 out]
    }
    frame 19 {
      # "DECREMENT_PROGRAM_FREQUENCY"
      n204 = Array To Cluster(array=w424) -> (cluster=w423:T4)
      n205 = Unbundle By Name(w423) -> ("DATA[0]"=w422:u8)
      n206 = Format Into String(format string="ProgramFrequencyIndex=%d\r\n", w422) -> (resulting string=w425:string)  [unwired: 2 in, 1 out]
    }
    frame 20 {
      # "INJECT_EVENT"
    }
    frame 21 {
      # "CHARGING_CONTROL"
      n207 = Array To Cluster(array=w439) -> (cluster=w438:T4)
      n208 = Unbundle By Name(w438) -> ("DATA[0]"=w433:u8, "DATA[1]"=w429:u8)
      n209 = And(x=240, y=w433) -> (x .and. y?=w435:i32)
      n210 = And(x=128, y=w433) -> (x .and. y?=w428:i32)
      n211 = And(x=w433, y=u8 15) -> (x .and. y?=w430:u8)
      n212 = case shown="48" w435 {
        tunnel: ["CHARGE_OFF-0" "CHARGE_PRE_CONDITION-1" "CHARGE_CONSTANT_CURRENT_FAST-2" "CHARGE_CONSTANT_CURRENT_SLOW-3" "CHARGE_COMPLETE-4" "CHARGE_ERROR-5" "CHARGE_CONSTANT_VOLTAGE_FAST-6" "CHARGE_CONSTANT_VOLTAGE_FAST-7"] -> w431
        frame 0, Default {
        }
        frame 16 {
        }
        frame 32 {
        }
        frame 48 {
        }
        frame 64 {
        }
        frame 80 {
        }
        frame 96 {
        }
        frame 112 {
        }
      }
      n213 = case shown="128" w428 {
        tunnel: ["NO" "YES"] -> w432
        frame 0, Default {
        }
        frame 128 {
          # "Charge Warning Bit Depricated"
        }
      }
      n214 = Format Into String(format string="ChargingState=%s\r\nChargeWarning=%s\r\nTemperatureLevel=%d\r\nIPG_ReceivedLevel=%d\r\n", w431, w432, w430, w429) -> (resulting string=w440:string)  [unwired: 2 in, 1 out]
    }
    frame 22 {
      # "GET_XPG_IDENTITY"
      n215 = Array Subset(array=w465, index=0, length=10) -> (w466:u8[])
      n216 = Array Subset(array=w465, index=10 ("length"), length=20) -> (w467:u8[])
      n217 = Array Subset(array=w465, index=30 ("length"), length=10) -> (w468:u8[])
      n218 = Byte Array To String(unsigned byte array=w466) -> (string=w458:string)
      n219 = Byte Array To String(unsigned byte array=w467) -> (string=w457:string)
      n220 = Byte Array To String(unsigned byte array=w468) -> (string=w456:string)
      n221 = Format Into String(format string="ModelNumber=%s\r\nSerialNumber=%s\r\nFirmwareVersion=%s\r\n", w458, w457, w456) -> (resulting string=w453:string)  [unwired: 2 in, 1 out]
      n222 = Search and Replace String(replace all?=TRUE ("replace all? (F)"), input string=w453, search string="\u0000") -> (result string=w452:string)  [unwired: 5 in, 3 out]
    }
    frame 23 {
      # "SET_XPG_IDENTITY"
    }
    frame 24 {
      # "RESTORE_PROGRAM_DEFAULTS"
    }
    frame 25 {
      w487 = "NO"
      w486 = "YES"
      # "GET_PROGRAM_DEFINITION"
      n223 = Index Array(array=w473, index=0) -> (element=w474:u8)
      n224 = Index Array(array=w473, index=2) -> (element=w508:u8)
      n225 = Index Array(array=w473, index=3) -> (element=w506:u8)
      n226 = Index Array(array=w473, index=28) -> (element=w478:u8)
      n227 = Index Array(array=w473, index=29) -> (element=w484:u8)
      n228 = for {
        N: 4 -> [_]
        tunnel: w473 -> [w565]
        shift-right: [w559] -> w477
        shift-left: "" -> [w560]
        i -> [w514]
        w524 = 8 ("index")
        w564 = 54 ("length")
        n229 = Multiply(x=w514, y=w564) -> (x*y=w562:i32)
        n230 = Add(x=30 ("index"), y=w562) -> (x+y=w563:i32)
        n231 = Array Subset(array=w565, index=w563, length=w564) -> (w521:u8[])
        n232 = case shown="3" w514 {
          tunnel: ["\r\n-- PULSE PA --\r\nPulseNamePA=%s\r\nAmplitudeLowLimitPA=%d\r\nAmplitudeStepPA=%d\r\nAmplitudeStepIndexPA=%d\r\nPulseWidthLowLimitPA=%d\r\nPulseWidthHighLimitPA=%d\r\nPulseWidthPA=%d\r\n%s" ("format string") "\r\n-- PULSE PB --\r\nPulseNamePB=%s\r\nAmplitudeLowLimitPB=%d\r\nAmplitudeStepPB=%d\r\nAmplitudeStepIndexPB=%d\r\nPulseWidthLowLimitPB=%d\r\nPulseWidthHighLimitPB=%d\r\nPulseWidthPB=%d\r\n%s" ("format string") "\r\n-- PULSE PC --\r\nPulseNamePC=%s\r\nAmplitudeLowLimitPC=%d\r\nAmplitudeStepPC=%d\r\nAmplitudeStepIndexPC=%d\r\nPulseWidthLowLimitPC=%d\r\nPulseWidthHighLimitPC=%d\r\nPulseWidthPC=%d\r\n%s" ("format string") "\r\n-- PULSE PD --\r\nPulseNamePD=%s\r\nAmplitudeLowLimitPD=%d\r\nAmplitudeStepPD=%d\r\nAmplitudeStepIndexPD=%d\r\nPulseWidthLowLimitPD=%d\r\nPulseWidthHighLimitPD=%d\r\nPulseWidthPD=%d\r\n%s" ("format string")] -> w556
          frame 0, Default {
          }
          frame 1 {
          }
          frame 2 {
          }
          frame 3 {
          }
        }
        n233 = Array Subset(array=w521, index=28, length=26) -> (w518:u8[])
        n234 = Array To Cluster(array=w521) -> (cluster=w553:T7)
        n235 = Unbundle By Name(w553) -> ("[16]"=w550:u8, "[17]"=w549:u8, "[18]"=w545:u8, "[19]"=w546:u8, "[20]"=w540:u8, "[21]"=w539:u8, "[22]"=w534:u8, "[23]"=w533:u8, "[24]"=w525:u8, "[25]"=w526:u8, "[26]"=w528:u8, "[27]"=w527:u8)
        n236 = Array Subset(array=w521, index=0, length=16) -> (w555:u8[])
        n237 = To Unsigned Word Integer(number=w549) -> (unsigned 16bit integer=w552:u16)
        n238 = To Unsigned Word Integer(number=w546) -> (unsigned 16bit integer=w548:u16)
        n239 = To Word Integer(number=w539) -> (16bit integer=w542:i16)
        n240 = To Unsigned Word Integer(number=w533) -> (unsigned 16bit integer=w537:u16)
        n241 = To Unsigned Word Integer(number=w526) -> (unsigned 16bit integer=w532:u16)
        n242 = To Unsigned Word Integer(number=w527) -> (unsigned 16bit integer=w530:u16)
        n243 = Byte Array To String(unsigned byte array=w555) -> (string=w554:string)
        n244 = Logical Shift(y=w524, x=w552) -> (x << y=w551:u16)
        n245 = Logical Shift(y=w524, x=w548) -> (x << y=w547:u16)
        n246 = Logical Shift(y=w524, x=w542) -> (x << y=w541:i16)
        n247 = Logical Shift(y=w524, x=w537) -> (x << y=w536:u16)
        n248 = Logical Shift(y=w524, x=w532) -> (x << y=w531:u16)
        n249 = Logical Shift(y=w524, x=w530) -> (x << y=w529:u16)
        n250 = Add(x=w550, y=w551) -> (x+y=w544:u16)
        n251 = Add(x=w545, y=w547) -> (x+y=w543:u16)
        n252 = Add(x=w540, y=w541) -> (x+y=w538:i16)
        n253 = Add(x=w534, y=w536) -> (x+y=w535:u16)
        n254 = Add(x=w525, y=w531) -> (x+y=w523:u16)
        n255 = Add(x=w528, y=w529) -> (x+y=w522:u16)
        n256 = for {
          N: 26 -> [_]
          tunnel: w518 -> [w577] mode=indexing
          shift-right: [w575] -> w516
          shift-left: "" -> [w576]
          tunnel: w514 -> [w570]
          i -> [w573]
          n257 = case shown="1" w570 {
            tunnel: ["ElectrodeAmpPercentPA[CH%02d]=%d\\r\\n" ("format string") "ElectrodeAmpPercentPB[CH%02d]=%d\\r\\n" ("format string") "ElectrodeAmpPercentPC[CH%02d]=%d\\r\\n" ("format string") "ElectrodeAmpPercentPD[CH%02d]=%d\\r\\n" ("format string")] -> w574
            frame 0, Default {
            }
            frame 1 {
            }
            frame 2 {
            }
            frame 3 {
            }
          }
          n258 = To Byte Integer(number=w577) -> (8bit integer=w571:i8)
          n259 = Increment(x=w573) -> (x+1=w572:i32)
          n260 = Format Into String(format string=w574, initial string=w576, w572, w571) -> (resulting string=w575:string)  [unwired: 1 in, 1 out]
        }
        n261 = Format Into String(format string=w556, initial string=w560, w554, w544, w543, w538, w535, w523, w522, w516) -> (resulting string=w559:string)  [unwired: 1 in, 1 out]
      }
      n262 = Array Subset(array=w473, index=4, length=16) -> (w505:u8[])
      n263 = Array Subset(array=w473, index=20, length=8) -> (w500:u8[])
      n264 = Number To Boolean Array(number=w484) -> (Boolean array=w493:bool[])
      n265 = Greater Than 0?(x=w508) -> (x > 0?=w496:bool)
      n266 = Greater Than 0?(x=w506) -> (x > 0?=w498:bool)
      n267 = Byte Array To String(unsigned byte array=w505) -> (string=w504:string)
      n268 = Array To Cluster(array=w493) -> (cluster=w492:T2)
      n269 = case shown="True" w496 {
        tunnel: ["NO" "YES"] -> w495
        frame False {
        }
        frame True {
        }
      }
      n270 = call <vilib>:"Trim Whitespace.vi"("string"=w504) -> ("trimmed string"=w472:string)  [unwired: 1 in]
      n271 = Unbundle By Name(w492) -> ("Boolean array[0]"=w491:bool, "Boolean array[1]"=w490:bool, "Boolean array[2]"=w489:bool, "Boolean array[3]"=w488:bool)
      n272 = case shown="False" w498 {
        tunnel: ["NO" "YES"] -> w497
        frame False {
        }
        frame True {
        }
      }
      n273 = for {
        shift-right: [w590] -> w499
        shift-left: "" -> [w591]
        tunnel: w500 -> [w592] mode=indexing
        i -> [w587]
        w588 = 8
        n274 = Multiply(x=w588, y=w587) -> (x*y=w586:i32)
        n275 = for {
          N: w588 -> [_]
          shift-right: [w599] -> w589
          shift-left: "" -> [w601]
          tunnel: w592 -> [w602]
          tunnel: w586 -> [w596]
          i -> [w597]
          n276 = Negate(x=w597) -> (-x=w603:i32)
          n277 = Add(x=w596, y=w597) -> (x+y=w595:i32)
          n278 = Logical Shift(y=w603, x=w602) -> (x << y=w604:u8)
          n279 = And(x=u8 1 ("width (-)"), y=w604) -> (x .and. y?=w594:u8)
          n280 = case shown="0, Default" w594 {
            tunnel: ["NO" "YES"] -> w598
            frame 0, Default {
            }
            frame 1 {
            }
          }
          n281 = Format Into String(format string="ProgramFreqTable[%02d]Allowed=%s\\r\\n", initial string=w601, w595, w598) -> (resulting string=w599:string)  [unwired: 1 in, 1 out]
        }
        n282 = Concatenate Strings(w591, w589) -> (w590:string)
      }
      n283 = Select(t=w486, s=w491, f=w487) -> (s? t:f=w483:string)
      n284 = Select(t=w486, s=w489, f=w487) -> (s? t:f=w481:string)
      n285 = Select(t=w486, s=w490, f=w487) -> (s? t:f=w482:string)
      n286 = Select(t=w486, s=w488, f=w487) -> (s? t:f=w480:string)
      n287 = Format Into String(format string="ProgramNumber=%d\r\nProgramDefined=%s\r\nProgramDisabled=%s\r\nProgramName=%s\r\n%sProgramFrequencyIndex=%d\r\nPA_Defined=%s\r\nPB_Defined=%s\r\nPC_Defined=%s\r\nPD_Defined=%s\r\n%s", w474, w495, w497, w472, w499, w478, w483, w482, w481, w480, w477) -> (resulting string=w512:string)  [unwired: 2 in, 1 out]
    }
    frame 26 {
      # "SET_PROGRAM_DEFINITION"
    }
    frame 27 {
      # "GET_PROGRAM_CONSTANTS"
      n288 = for {
        N: 64 -> [_]
        shift-right: [w630] -> w609
        shift-left: "" -> [w631]
        tunnel: w610 -> [w627]
        i -> [w625]
        w624 = 2 ("index")
        n289 = Multiply(x=w625, y=w624) -> (x*y=w626:i32)
        n290 = Add(x=w626, y=w624) -> (x+y=w623:i32)
        n291 = Array Subset(array=w627, index=w623, length=2) -> (w622:u8[])
        n292 = Array To Cluster(array=w622) -> (cluster=w621:cluster{"[0]":u8, "[1]":u8})
        n293 = Unbundle(w621) -> ("[0]"=w617:u8, "[1]"=w616:u8)
        n294 = To Unsigned Word Integer(number=w616) -> (unsigned 16bit integer=w620:u16)
        n295 = Logical Shift(y=i8 8, x=w620) -> (x << y=w618:u16)
        n296 = Add(x=w617, y=w618) -> (x+y=w615:u16)
        n297 = Format Into String(format string="ProgramFrequencies[%02d]=%d\r\n", initial string=w631, w625, w615) -> (resulting string=w630:string)  [unwired: 1 in, 1 out]
      }
      n298 = Format Into String(format string="%s", w609) -> (resulting string=w613:string)  [unwired: 2 in, 1 out]
    }
    frame 28 {
      # "SET_PROGRAM_CONSTANTS"
    }
    frame 29 {
      w641 = "NO"
      w642 = "YES"
      # "Convert MS DateTime\nto LV DateTime"
      # "GET_CONFIGURABLE_DEVICE_PARAMETERS"
      n299 = Array To Cluster(array=w635) -> (cluster=w665:T8)
      n300 = Unbundle By Name(w665) -> ("DATA[0]"=w699:u8, "DATA[1]"=w697:u8, "DATA[2]"=w695:u8, "DATA[3]"=w694:u8, "DATA[4]"=w693:u8, "DATA[5]"=w690:u8, "DATA[6]"=w689:u8, "DATA[7]"=w688:u8, "DATA[8]"=w687:u8, "DATA[9]"=w684:u8, "DATA[10]"=w683:u8, "DATA[11]"=w682:u8)
      n301 = Unbundle By Name(w665) -> ("DATA[42]"=w662:u8, "DATA[43]"=w661:u8, "DATA[44]"=w658:u8, "DATA[45]"=w657:u8, "DATA[46]"=w646:u8)
      n302 = Index Array(array=w635, index=56) -> (element=w634:u8)
      n303 = Array Subset(array=w635, index=48, length=8) -> (w672:u8[])
      n304 = Array Subset(array=w635, index=12, length=30) -> (w667:u8[])
      n305 = for {
        tunnel: w672 -> [w709] mode=indexing
        shift-right: [w703] -> w677
        shift-left: u64 0 ("y") -> [w704]
        tunnel: i8 8 ("y") -> [w707]
        i -> [w708]
        n306 = To Unsigned Quad Integer(1:w709) -> (0:w702:u64)
        n307 = Multiply(x=w707, y=w708) -> (x*y=w706:i32)
        n308 = Logical Shift(y=w706, x=w702) -> (x << y=w705:u64)
        n309 = Add(x=w704, y=w705) -> (x+y=w703:u64)
      }
      n310 = Greater Than 0?(x=w699) -> (x > 0?=w698:bool)
      n311 = Greater Than 0?(x=w693) -> (x > 0?=w692:bool)
      n312 = Greater Than 0?(x=w687) -> (x > 0?=w686:bool)
      n313 = Byte Array To String(unsigned byte array=w667) -> (string=w666:string)
      n314 = To Unsigned Word Integer(number=w661) -> (unsigned 16bit integer=w664:u16)
      n315 = Number To Boolean Array(number=w657) -> (Boolean array=w655:bool[])
      n316 = Number To Boolean Array(number=w646) -> (Boolean array=w647:bool[])
      n317 = Logical Shift(y=i8 8, x=w664) -> (x << y=w663:u16)
      n318 = Array To Cluster(array=w655) -> (cluster=w656:T2)
      n319 = Array To Cluster(array=w647) -> (cluster=w648:T2)
      n320 = Add(x=w662, y=w663) -> (x+y=w659:u16)
      n321 = Unbundle By Name(w656) -> ("Boolean array[0]"=w653:bool, "Boolean array[1]"=w654:bool, "Boolean array[2]"=w651:bool)
      n322 = Unbundle By Name(w648) -> ("Boolean array[0]"=w643:bool, "Boolean array[1]"=w645:bool, "Boolean array[2]"=w644:bool)
      n323 = Multiply(x=u64 1904 ("y"), y=u64 31556926) -> (x*y=w675:u64)
      n324 = Quotient & Remainder(x=w677, y=u64 10000000) -> (floor(x/y)=w633:u64)  [unwired: 1 out]
      n325 = Subtract(x=w633, y=w675) -> (x-y=w673:u64)
      n326 = Format Date/Time String(seconds (now)=w673, UTC format=FALSE) -> (date/time string=w637:string)  [unwired: 1 in]
      n327 = Select(t=w642, s=w692, f=w641) -> (s? t:f=w691:string)
      n328 = Select(t=w642, s=w653, f=w641) -> (s? t:f=w652:string)
      n329 = Select(t=w642, s=w651, f=w641) -> (s? t:f=w649:string)
      n330 = Select(t=w642, s=w645, f=w641) -> (s? t:f=w639:string)
      n331 = Select(t=w642, s=w698, f=w641) -> (s? t:f=w696:string)
      n332 = Select(t=w642, s=w686, f=w641) -> (s? t:f=w685:string)
      n333 = Select(t=w642, s=w654, f=w641) -> (s? t:f=w650:string)
      n334 = Select(t=w642, s=w643, f=w641) -> (s? t:f=w640:string)
      n335 = Select(t=w642, s=w644, f=w641) -> (s? t:f=w638:string)
      n336 = Format Into String(format string="PPC_Enabled=%s\r\nPPC_EXID[0]=0x%02x\r\nPPC_EXID[1]=0x%02x\r\nPPC_EXID[2]=0x%02x\r\nPOP1_Enabled=%s\r\nPOP1_EXID[0]=0x%02x\r\nPOP1_EXID[1]=0x%02x\r\nPOP1_EXID[2]=0x%02x\r\nPOP2_Enabled=%s\r\nPOP2_EXID[0]=0x%02x\r\nPOP2_EXID[1]=0x%02x\r\nPOP2_EXID[2]=0x%02x\r\nPPC_Text=%s\r\nPulseWidthStep=%d\r\nAmplitudeSteps=%d\r\nPPC_AllowIndividualPulseAmplMod=%s\r\nPPC_AllowIndividualPulseWidthMod=%s\r\nPPC_AllowProgramFreqMod=%s\r\nIPG_MagnetOptions_Behavior_A_Enabled=%s\r\nIPG_MagnetOptions_Behavior_B_Enabled=%s\r\nIPG_MagnetOptions_Behavior_C_Enabled=%s\r\nImplantDateTime=%s\r\nReplacementIntervalMonths=%d\r\n", w696, w697, w695, w694, w691, w690, w689, w688, w685, w684, w683, w682, w666, w659, w658, w652, w650, w649, w640, w639, w638, w637, w634) -> (resulting string=w700:string)  [unwired: 2 in, 1 out]
    }
    frame 30 {
      # "SET_CONFIGURABLE_DEVICE_PARAMETERS"
    }
    frame 31 {
      w719 = "NO"
      w718 = "YES"
      w764 = i8 8 ("y")
      # "GET_PULSE_CONSTANTS"
      n337 = Array To Cluster(array=w785) -> (cluster=w786:T9)
      n338 = Unbundle By Name(w786) -> ("DATA[0]"=w763:u8, "DATA[1]"=w743:u8, "DATA[2]"=w762:u8, "DATA[3]"=w711:u8, "DATA[4]"=w761:u8, "DATA[5]"=w744:u8, "DATA[6]"=w760:u8, "DATA[7]"=w745:u8, "DATA[8]"=w759:u8, "DATA[9]"=w746:u8, "DATA[10]"=w758:u8, "DATA[11]"=w747:u8, "DATA[12]"=w757:u8, "DATA[13]"=w748:u8, "DATA[14]"=w756:u8, "DATA[15]"=w749:u8, "DATA[16]"=w755:u8, "DATA[17]"=w750:u8, "DATA[18]"=w754:u8, "DATA[19]"=w751:u8, "DATA[20]"=w753:u8, "DATA[21]"=w752:u8, "DATA[22]"=w717:u8, "DATA[23]"=w716:u8)
      n339 = To Unsigned Word Integer(number=w743) -> (unsigned 16bit integer=w788:u16)
      n340 = To Unsigned Word Integer(number=w711) -> (unsigned 16bit integer=w784:u16)
      n341 = To Unsigned Word Integer(number=w744) -> (unsigned 16bit integer=w782:u16)
      n342 = To Unsigned Word Integer(number=w745) -> (unsigned 16bit integer=w780:u16)
      n343 = To Unsigned Word Integer(number=w746) -> (unsigned 16bit integer=w778:u16)
      n344 = To Unsigned Word Integer(number=w747) -> (unsigned 16bit integer=w776:u16)
      n345 = To Unsigned Word Integer(number=w748) -> (unsigned 16bit integer=w774:u16)
      n346 = To Unsigned Word Integer(number=w749) -> (unsigned 16bit integer=w772:u16)
      n347 = To Unsigned Word Integer(number=w750) -> (unsigned 16bit integer=w770:u16)
      n348 = To Unsigned Word Integer(number=w751) -> (unsigned 16bit integer=w768:u16)
      n349 = To Unsigned Word Integer(number=w752) -> (unsigned 16bit integer=w766:u16)
      n350 = Logical Shift(y=w764, x=w788) -> (x << y=w787:u16)
      n351 = Logical Shift(y=w764, x=w784) -> (x << y=w783:u16)
      n352 = Logical Shift(y=w764, x=w782) -> (x << y=w781:u16)
      n353 = Logical Shift(y=w764, x=w780) -> (x << y=w779:u16)
      n354 = Logical Shift(y=w764, x=w778) -> (x << y=w777:u16)
      n355 = Logical Shift(y=w764, x=w776) -> (x << y=w775:u16)
      n356 = Logical Shift(y=w764, x=w774) -> (x << y=w773:u16)
      n357 = Logical Shift(y=w764, x=w772) -> (x << y=w771:u16)
      n358 = Logical Shift(y=w764, x=w770) -> (x << y=w769:u16)
      n359 = Logical Shift(y=w764, x=w768) -> (x << y=w767:u16)
      n360 = Logical Shift(y=w764, x=w766) -> (x << y=w765:u16)
      n361 = Add(x=w763, y=w787) -> (x+y=w742:u16)
      n362 = Add(x=w762, y=w783) -> (x+y=w741:u16)
      n363 = Add(x=w761, y=w781) -> (x+y=w740:u16)
      n364 = Add(x=w760, y=w779) -> (x+y=w739:u16)
      n365 = Add(x=w759, y=w777) -> (x+y=w738:u16)
      n366 = Add(x=w758, y=w775) -> (x+y=w737:u16)
      n367 = Add(x=w757, y=w773) -> (x+y=w736:u16)
      n368 = Add(x=w756, y=w771) -> (x+y=w735:u16)
      n369 = Add(x=w755, y=w769) -> (x+y=w734:u16)
      n370 = Add(x=w754, y=w767) -> (x+y=w733:u16)
      n371 = Add(x=w753, y=w765) -> (x+y=w720:u16)
      n372 = Number To Boolean Array(number=w733) -> (Boolean array=w732:bool[])
      n373 = Array To Cluster(array=w732) -> (cluster=w731:T10)
      n374 = Unbundle By Name(w731) -> ("Boolean array[0]"=w730:bool, "Boolean array[1]"=w729:bool, "Boolean array[2]"=w728:bool, "Boolean array[3]"=w723:bool, "Boolean array[4]"=w722:bool)
      n375 = Greater Than 0?(x=w717) -> (x > 0?=w715:bool)
      n376 = Greater Than 0?(x=w716) -> (x > 0?=w714:bool)
      n377 = Select(t=w718, s=w730, f=w719) -> (s? t:f=w727:string)
      n378 = Select(t=w718, s=w728, f=w719) -> (s? t:f=w725:string)
      n379 = Select(t=w718, s=w722, f=w719) -> (s? t:f=w721:string)
      n380 = Select(t=w718, s=w714, f=w719) -> (s? t:f=w712:string)
      n381 = Select(t=w718, s=w729, f=w719) -> (s? t:f=w726:string)
      n382 = Select(t=w718, s=w723, f=w719) -> (s? t:f=w724:string)
      n383 = Select(t=w718, s=w715, f=w719) -> (s? t:f=w713:string)
      n384 = Format Into String(format string="PassiveInterphaseDelay=%d\r\nPassiveRecoveryWidth=%d\r\nPassiveRecoveryHoldoff=%d\r\nPassiveCBCWidth=%d\r\nPassiveCBCHoldoff=%d\r\nActiveInterphaseDelay=%d\r\nActiveRecoveryHoldoff=%d\r\nActiveCBCWidth=%d\r\nActiveCBCHoldoff=%d\r\nKrec[1]Enabled=%s\r\nKrec[2]Enabled=%s\r\nKrec[3]Enabled=%s\r\nKrec[4]Enabled=%s\r\nKrec[5]Enabled=%s\r\nIncrementLockoutMsecs=%d\r\nStimPhasePSDisableActive=%s\r\nUncontrolledSourceSinkEnabled=%s\r\n", w742, w741, w740, w739, w738, w737, w736, w735, w734, w727, w726, w725, w724, w721, w720, w713, w712) -> (resulting string=w789:string)  [unwired: 2 in, 1 out]
    }
    frame 32 {
      # "SET_PULSE_CONSTANTS"
    }
    frame 33 {
      # "GET_LEAD_LIMITS"
      n385 = for {
        N: 26 -> [_]
        shift-right: [w837] -> w792
        shift-left: "" -> [w838]
        tunnel: w794 -> [w834]
        i -> [w832]
        n386 = Multiply(x=w832, y=2 ("index")) -> (x*y=w833:i32)
        n387 = Add(x=w833, y=52) -> (x+y=w830:i32)
        n388 = Array Subset(array=w834, index=w830, length=2) -> (w829:u8[])
        n389 = Increment(x=w832) -> (x+1=w820:i32)
        n390 = Array To Cluster(array=w829) -> (cluster=w828:cluster{"[0]":u8, "[1]":u8})
        n391 = Unbundle(w828) -> ("[0]"=w824:u8, "[1]"=w823:u8)
        n392 = To Unsigned Word Integer(number=w823) -> (unsigned 16bit integer=w827:u16)
        n393 = Logical Shift(y=i8 8, x=w827) -> (x << y=w825:u16)
        n394 = Add(x=w824, y=w825) -> (x+y=w822:u16)
        n395 = Format Into String(format string="chargeLimit[%02d]=%d\r\n", initial string=w838, w820, w822) -> (resulting string=w837:string)  [unwired: 1 in, 1 out]
      }
      n396 = for {
        N: 26 -> [_]
        shift-right: [w818] -> w793
        shift-left: "" -> [w819]
        tunnel: w794 -> [w815]
        i -> [w813]
        n397 = Multiply(x=w813, y=2 ("index")) -> (x*y=w814:i32)
        n398 = Add(x=w814, y=0) -> (x+y=w811:i32)
        n399 = Array Subset(array=w815, index=w811, length=2) -> (w810:u8[])
        n400 = Increment(x=w813) -> (x+1=w801:i32)
        n401 = Array To Cluster(array=w810) -> (cluster=w809:cluster{"[0]":u8, "[1]":u8})
        n402 = Unbundle(w809) -> ("[0]"=w805:u8, "[1]"=w804:u8)
        n403 = To Unsigned Word Integer(number=w804) -> (unsigned 16bit integer=w808:u16)
        n404 = Logical Shift(y=i8 8, x=w808) -> (x << y=w806:u16)
        n405 = Add(x=w805, y=w806) -> (x+y=w803:u16)
        n406 = Format Into String(format string="currentLimit[%02d]=%d\r\n", initial string=w819, w801, w803) -> (resulting string=w818:string)  [unwired: 1 in, 1 out]
      }
      n407 = Format Into String(format string="%s%s", w793, w792) -> (resulting string=w799:string)  [unwired: 2 in, 1 out]
    }
    frame 34 {
      # "SET_LEAD_LIMITS"
    }
    frame 35 {
      # "GET_CHANNEL_CALIBRATIONS"
      n408 = Split 1D Array(array=w852, index=2) -> (first subarray=w841:u8[], second subarray=w850:u8[])
      n409 = for {
        N: 26 -> [_]
        shift-right: [w895] -> w849
        shift-left: "" -> [w896]
        tunnel: w850 -> [w892]
        i -> [w890]
        n410 = Multiply(x=w890, y=2 ("index")) -> (x*y=w891:i32)
        n411 = Add(x=w891, y=52) -> (x+y=w888:i32)
        n412 = Array Subset(array=w892, index=w888, length=2) -> (w887:u8[])
        n413 = Increment(x=w890) -> (x+1=w878:i32)
        n414 = Array To Cluster(array=w887) -> (cluster=w886:cluster{"[0]":u8, "[1]":u8})
        n415 = Unbundle(w886) -> ("[0]"=w882:u8, "[1]"=w881:u8)
        n416 = To Unsigned Word Integer(number=w881) -> (unsigned 16bit integer=w885:u16)
        n417 = Logical Shift(y=i8 8, x=w885) -> (x << y=w883:u16)
        n418 = Add(x=w882, y=w883) -> (x+y=w880:u16)
        n419 = Format Into String(format string="channelCalSinking[%02d]=%d\r\n", initial string=w896, w878, w880) -> (resulting string=w895:string)  [unwired: 1 in, 1 out]
      }
      n420 = for {
        N: 26 -> [_]
        shift-right: [w876] -> w848
        shift-left: "" -> [w877]
        tunnel: w850 -> [w873]
        i -> [w871]
        n421 = Multiply(x=w871, y=2 ("index")) -> (x*y=w872:i32)
        n422 = Add(x=w872, y=0) -> (x+y=w869:i32)
        n423 = Array Subset(array=w873, index=w869, length=2) -> (w868:u8[])
        n424 = Increment(x=w871) -> (x+1=w859:i32)
        n425 = Array To Cluster(array=w868) -> (cluster=w867:cluster{"[0]":u8, "[1]":u8})
        n426 = Unbundle(w867) -> ("[0]"=w863:u8, "[1]"=w862:u8)
        n427 = To Unsigned Word Integer(number=w862) -> (unsigned 16bit integer=w866:u16)
        n428 = Logical Shift(y=i8 8, x=w866) -> (x << y=w864:u16)
        n429 = Add(x=w863, y=w864) -> (x+y=w861:u16)
        n430 = Format Into String(format string="channelCalSourcing[%02d]=%d\r\n", initial string=w877, w859, w861) -> (resulting string=w876:string)  [unwired: 1 in, 1 out]
      }
      n431 = Array To Cluster(array=w841) -> (cluster=w847:cluster{"[0]":u8, "[1]":u8})
      n432 = Unbundle(w847) -> ("[0]"=w843:u8, "[1]"=w842:u8)
      n433 = To Unsigned Word Integer(number=w842) -> (unsigned 16bit integer=w846:u16)
      n434 = Logical Shift(y=i8 8, x=w846) -> (x << y=w844:u16)
      n435 = Add(x=w843, y=w844) -> (x+y=w840:u16)
      n436 = Format Into String(format string="Index=%d\r\n%s%s", w840, w848, w849) -> (resulting string=w857:string)  [unwired: 2 in, 1 out]
    }
    frame 36 {
      # "SET_CHANNEL_CALIBRATIONS"
    }
    frame 43 {
      # "GET_STIM_ASIC_HV_CALIBRATIONS"
      n437 = for {
        N: 64 -> [_]
        shift-right: [w920] -> w898
        shift-left: "" -> [w921]
        tunnel: w899 -> [w917]
        i -> [w915]
        n438 = Multiply(x=w915, y=2 ("index")) -> (x*y=w916:i32)
        n439 = Add(x=w916, y=0) -> (x+y=w913:i32)
        n440 = Array Subset(array=w917, index=w913, length=2) -> (w912:u8[])
        n441 = Array To Cluster(array=w912) -> (cluster=w911:cluster{"[0]":u8, "[1]":u8})
        n442 = Unbundle(w911) -> ("[0]"=w907:u8, "[1]"=w906:u8)
        n443 = To Unsigned Word Integer(number=w906) -> (unsigned 16bit integer=w910:u16)
        n444 = Logical Shift(y=i8 8, x=w910) -> (x << y=w908:u16)
        n445 = Add(x=w907, y=w908) -> (x+y=w905:u16)
        n446 = Format Into String(format string="Stim_ASIC_HV_mV_Output[%02d]=%d\r\n", initial string=w921, w915, w905) -> (resulting string=w920:string)  [unwired: 1 in, 1 out]
      }
      n447 = Format Into String(format string="%s", w898) -> (resulting string=w902:string)  [unwired: 2 in, 1 out]
    }
    frame 44 {
      # "SET_STIM_ASIC_HV_CALIBRATIONS"
    }
    frame 47 {
      # "GET_CP_DATA"
      n448 = for {
        N: 256 -> [_]
        shift-right: [w933] -> w924
        shift-left: "" -> [w934]
        tunnel: w925 -> [w930] mode=indexing
        tunnel: [w930] -> w923 mode=indexing
        i -> [w931]
        n449 = Format Into String(format string="CP_Data[%03d]=0x%02x\r\n", initial string=w934, w931, w930) -> (resulting string=w933:string)  [unwired: 1 in, 1 out]
      }
      "CP_DATA" <- w923
      n450 = Format Into String(format string="%s", w924) -> (resulting string=w928:string)  [unwired: 2 in, 1 out]
    }
    frame 48 {
      # "SET_CP_DATA"
    }
    frame 49 {
      # "CLEAR_LOG"
    }
    frame 50 {
      w951 = string[][] [["0", " The null event."], ["1001", " An unintended reset occurred."], ["1002", " A watchdog reset occurred."], ["1003", " An error was detected during a voltage check."], ["1004", " An error was detected during a temperature check."], ["1005", " A timing error was detected during clock verification."], ["1006", " A timing error was detected during pulse cycle verification"], ["1010", " A Stimulation Data Read-back error was detected."], ["1011", " The diagnostic memory check detected corruption of the Stimulation Program Definition."], ["1012", " The diagnostic memory check detected corruption of the Active Stimulation Settings."], ["1013", " The diagnostic memory check detected corruption of the MICS identity information."], ["1014", " The diagnostic memory check detected corruption of the Program Constants."], ["1015", " The diagnostic memory check detected corruption of the Pulse Constants."], ["1016", " The diagnostic memory check detected corruption of the Channel Calibration."], ["1017", " The diagnostic memory check detected corruption of the Lead Information."], ["1018", " The diagnostic memory check detected corruption of the Configurable Device Parameters."], ["1019", " The diagnostic memory check detected corruption of the General Calibration Data."], ["1020", " The Stimulation System trim list is corrupted."], ["1021", " The Power System trim list is corrupted."], ["1022", " The Radio trim list is corrupted."], ["1023", " The Program Data Integrity check failed"], ["1024", " The diagnostic memory check detected corruption of the High Voltage Calibration"], ["1025", " The diagnostic memory check detected corruption of the Background Impedance Parameters"], ["1026", " The diagnostic memory check detected corruption of the Ramp Time"], ["1030", " A Brownout was detected during Stimulation."], ["1040", " The pulse guard tripped."], ["1041", " A stimulation system parity error was detected."], ["1042", " A stimulation system sequencing error"], ["1043", " A stimulation system address error"], ["1044", " A stimulation system register valid error"], ["1045", " A stimulation system write protect error"], ["1050", " The Impedance Measurement diagnostics detected an Open Circuit Condition."], ["1051", " The Background Stimulation Output check detected a Faulty Channel."], ["1052", " The Output Capacitor check detected a Faulty Capacitor."], ["1053", " Background Impedance Measurement failed"], ["1054", " The Check Densities routine failed"], ["1055", " The Stimulation hardware didn't power up or initialize correctly"], ["1056", " Basic Output Check failed"], ["1057", " Diagnostic Output Check failed"], ["1060", " The Thermistor Diagnostic detects a fault in the temperature measurement circuit"], ["1070", " The Log Module detected a corrupt Event Log data structure in this Log"], ["1071", " The software has exceeded its stack limitations"], ["1072", " The software has detected a queue overflow"], ["1080", " Unknown error has been published"], ["1081", " System restarted after coming out of reset"], ["1082", " System restarted after receiving unknown interrupt"], ["1083", " System restarted for unknown reasons"], ["1090", " Test stim range check failed"], ["1091", " Retrieving a program failed"], ["1092", " Stim auto-waveform failed"], ["1093", " Compliance voltage calculation indicates voltage higher than is available"], ["1094", " Stim high voltage DAC initialization failed"], ["1095", " Stim period check failed"], ["1096", " Stim calculated a pulse width - frequency conflict"], ["2001", " Embed timestamp low bytes in log"], ["2002", " Mark location in log"], ["2003", " System is powered up or coming out of a reset"], ["2004", " CP has been connected to the system"], ["2005", " Embed timestamp high bytes in log"], ["2006", " MICS Connection established data includes channel number"], ["2007", " MICS has been disconnected by the software"], ["2008", " MICS has been shutdown"], ["2009", " MICS transmit/receive has been aborted"], ["2010", " MICS driver has been initialized"], ["2011", " MICS connection has been lost"], ["2012", " MICS radio failure"], ["2013", " MICS radio is ready"], ["2014", " MICS link is ready"], ["2016", " MICS MAC Command Timeout"], ["2017", " MICS Watchdog Timeout"], ["2018", " MICS Housekeeping Abort Link"], ["2020", " Charging of the battery has been initiated"], ["2021", " Battery has been charged to full capacity"], ["2022", " Battery charging has been interrupted prior to being fully charged"], ["2023", " Charger has been detected"], ["2024", " Charger has been removed"], ["2025", " Charging has been aborted due to high temperature"], ["2026", " Charging has been aborted due to insufficient voltage rise"], ["2027", " Charging has been aborted due to error"], ["2028", " Charging has been disconnected from the system"], ["2029", " Stimulation was stopped due to low battery"], ["2030", " Stimulation was stopped due to power down"], ["2031", " Stimulation was stopped due to an error"], ["2032", " Charging was stopped due to overvoltage error"], ["2033", " Charging was switched to C8 because of critical temperature"], ["2034", " Charging was switched to the mode specified"], ["2040", " Stimulation was stopped to radio session closing"], ["2041", " Pairing information was changed via radio"], ["2042", " Pairing information was changed via charging system"], ["2050", " Calibration data restored from backup"], ["2051", " Program or Pulse constants data has been repaired"], ["2052", " High Voltage Calibration data was restored from backup"], ["2053", " General Calibration data was restored from backup"], ["2054", " System Information Data was restored from backup copy"], ["2055", " Stimulation configuration trim list data was restored from backup"], ["2056", " Radio configuration trim list data was restored from backup"], ["2057", " Default background impedance parameters have been restored"], ["2058", " Power configuration trim list data was restored from backup"], ["2059", " Configurable device parameters was restored from backup"], ["2060", " Ramp time was restored from backup"], ["2070", " The command received was not supported"], ["2071", " Stimulation was stopped"], ["2072", " Patient stimulation was started"], ["2073", " Trial stimulation was started"], ["2074", " Test stimulation was started"], ["2075", " System was commanded into storage mode"], ["2076", " Patient Program was selected"], ["2077", " Program amplitude was incremented"], ["2078", " Pulse amplitude was incremented"], ["2079", " Program frequency was set"], ["2080", " Active Program Settings were restored to default values"], ["2081", " System was commanded to reset"], ["2082", " Impedance measurement was requested"], ["2083", " Log was requested to be cleared"], ["2084", " Trial Stimulation parameters were modified"], ["2089", " Test Stimulation parameters were modified"], ["2090", " Program amplitude was decremented"], ["2100", " Patient stimulation was started via magnet"], ["2101", " Patient stimulation was stopped via magnet"], ["2102", " System is about the powered down via magnet"], ["2110", " Stimulation is stopped via charging system command"], ["2120", " Error log was read"], ["2121", " Event log was read"], ["2122", " PPC Constants were queried"], ["2123", " Program names were queried"], ["2124", " Program constants were queried"], ["2125", " System Identity information was queried"], ["2126", " General calibration parameters were queried"], ["2127", " Charging went from current mode to voltage mode counter was queried"], ["2128", " Charging was done to completion counter was queried"], ["2129", " Storage mode counter was queried"], ["2130", " Channel calibration values were queried"], ["2131", " High Voltage calibration values were queried"], ["2132", " Trim list values were queried"], ["2133", " Battery diagnostic information was queried"], ["2134", " Background impedance diagnostic information was queried"], ["2135", " Output capacitor check diagnostic information was queried"], ["2136", " Thermistor diagnostic information was queried"], ["2137", " Program definition was queried"], ["2138", " Pulse constants were queried"], ["2139", " Configuration device parameters were queried"], ["2140", " Pulse widths were queried"], ["2141", " Program frequency was queried"], ["2142", " POP Constants were queried"], ["2143", " Lead limits were queried"], ["2144", " Clinician Programmer data was queried"], ["2145", " Ramp Time was queried"], ["2146", " Trial Stimulation parameters were queried"], ["2147", " Program run time was queried"], ["2148", " Direct memory read was performed"], ["2149", " Background impedance parameters were queried"], ["2201", " System Identity Information changed"], ["2202", " General calibration data changed"], ["2203", " Charging mode change counter was reset"], ["2204", " Charging completed counter was reset"], ["2205", " Storage mode counter was reset"], ["2206", " Channel calibration was changed"], ["2207", " High Voltage calibration was changed"], ["2208", " Stimulation configuration trim list was changed"], ["2209", " Radio configuration trim list was changed"], ["2210", " Program definition was changed"], ["2211", " Program constants were changed"], ["2212", " Pulse constants were changed"], ["2213", " Config device parameters were changed"], ["2214", " Lead limits were changed"], ["2215", " Clinician Program data was changed"], ["2216", " Ramp Time was changed"], ["2217", " Program Time was reset"], ["2218", " Direct write to memory was requested"], ["2219", " Background Impedance Parameters were changed"], ["2220", " System Error was detected"], ["2221", " Charging Error was detected"], ["2222", " Power configuration trim list was changed"], ["2300", " Diagnostic log of vrect and temperature during charging"], ["2301", " Diagnostic log of temperature data during charging"], ["2302", " Diagnostic log of battery adc counts during charging"], ["2303", " The MICS ISR was unable to clear an interrupt bit. Data contains (lsb) after processing irq stat2 register after processing irq stat 1 register before processing irq stat 2 register before processing irq stat 1 register (msb)"], ["2304", " The MICS driver failed to write to a register via SPI. Data contains (lsb) read register value written register value register address (msb)"], ["2305", " The MSP430 VLO was calibrated and is running at the specified frequency"], ["2308", " E_LOG_MICS_RSSI"], ["2400", " A MICS Command was received token is logged"], ["2401", " A MICS Response was sent token is logged"], ["2402", " A MICS Packet was dumped"], ["2403", " A MICS Command was received from an unpaired programmer"], ["2404", " A MICS Command with an invalid token was received"], ["2405", " A MICS Command was received but the checksum failed"], ["2406", " A MICSPAD Timeout occurred waiting for an intermediate block"], ["2407", " A MICS Session was closed by the MICS PAD"], ["2450", " A byte was received over TETS data has byte"], ["2451", " A valid TETS command was received data has command number"], ["2452", " A response is being sent over TETS"], ["2453", " A byte was sent over TETS data has byte"], ["2454", " TETS command was rejected because message not formatted correctly"], ["2455", " A timeout occurred while sending or receving data bytes"], ["2500", "Debug"], ["", "PULSE_GUARD_MEMORY_ERROR"], ["", "PULSE_GUARD_CLOCK_ERROR"], ["", "PULSE_GUARD_UNKNOWN_ERROR"]]  # Event descriptions from .h file
      # "( Mark's updates )\nERIK UPDATE"
      # "READ_LOG"
      n451 = Array To Cluster(array=w954) -> (cluster=w938:T6)
      n452 = Unbundle By Name(w938) -> ("DATA[0]"=w939:u8, "DATA[1]"=w946:u8, "DATA[7]"=w942:u8, "DATA[6]"=w943:u8, "DATA[5]"=w944:u8, "DATA[4]"=w945:u8)
      n453 = Join Numbers(hi=w942, lo=w943) -> ((hi.lo)=w941:u16)
      n454 = Join Numbers(hi=w944, lo=w945) -> ((hi.lo)=w940:u16)
      n455 = Join Numbers(hi=w941, lo=w940) -> ((hi.lo)=w952:u32)
      n456 = Array Subset(array=w954, index=8) -> (w947:u8[])  [unwired: 1 in]
      n457 = for {
        N: w946 -> [_]
        tunnel: w947 -> [w986]
        tunnel: 10 ("index") -> [w971]
        shift-right: [w983] -> w953
        shift-left: "" -> [w982]
        tunnel: w951 -> [w961]
        i -> [w970]
        n458 = Index Array(array=w961, index (col) #1=0 ("disabled index (col)"), index (col) #2=1 ("disabled index (col)")) -> (element #1=w964:string[], element #2=w957:string[])  [unwired: 2 in]
        n459 = Multiply(x=w970, y=w971) -> (x*y=w966:i32)
        n460 = Array Subset(array=w986, index=w966, length=w971) -> (w985:u8[])
        n461 = Array To Cluster(array=w985) -> (cluster=w984:T11)
        n462 = Unbundle By Name(w984) -> ("[3]"=w978:u8, "[2]"=w977:u8, "[1]"=w976:u8, "[0]"=w975:u8, "[5]"=w968:u8, "[4]"=w969:u8, "[6]"=w960:u8, "[7]"=w973:u8, "[8]"=w972:u8, "[9]"=w967:u8)
        n463 = Join Numbers(hi=w968, lo=w969) -> ((hi.lo)=w956:u16)
        n464 = Join Numbers(hi=w978, lo=w977) -> ((hi.lo)=w979:u16)
        n465 = Join Numbers(hi=w976, lo=w975) -> ((hi.lo)=w980:u16)
        n466 = Number To Decimal String(number=w956) -> (decimal integer string=w963:string)  [unwired: 1 in]
        n467 = Join Numbers(hi=w979, lo=w980) -> ((hi.lo)=w974:u32)
        n468 = Search 1D Array(1D array=w964, element=w963) -> (index of element=w962:i32)  [unwired: 1 in]
        n469 = Index Array(array=w957, index=w962) -> (element=w959:string)
        n470 = Format Into String(format string="\\r\\nTimestamp=%d\\r\\nEvent=%d\\r\\nDescription=%s\\r\\nEventData[0]=%02x\\r\\nEventData[1]=%02x\\r\\nEventData[2]=%02x\\r\\nEventData[3]=%02x\\r\\n", initial string=w982, w974, w956, w959, w960, w973, w972, w967) -> (resulting string=w983:string)  [unwired: 1 in, 1 out]
      }
      n471 = Format Into String(format string="LogNum=%d\r\nCount=%d\r\nSerial=%d\r\n%s", w939, w946, w952, w953) -> (resulting string=w955:string)  [unwired: 2 in, 1 out]
    }
    frame 51 {
      # "APPEND_LOG"
      n472 = Array To Cluster(array=w988) -> (cluster=w989:T6)
      n473 = disable-structure shown="Enabled" {
        disable-tunnel: w989 -> [w999 w1001]
        disable-tunnel: [w992 w1000] -> w987
        frame Enabled {
          n474 = Unbundle By Name(w999) -> ("DATA[3]"=w998:u8, "DATA[2]"=w997:u8, "DATA[1]"=w996:u8, "DATA[0]"=w995:u8)
          n475 = Join Numbers(hi=w998, lo=w997) -> ((hi.lo)=w994:u16)
          n476 = Join Numbers(hi=w996, lo=w995) -> ((hi.lo)=w993:u16)
          n477 = Join Numbers(hi=w994, lo=w993) -> ((hi.lo)=w992:u32)
        }
        frame Disabled {
          n478 = Unbundle By Name(w1001) -> ("DATA[0]"=w1000:u8)
        }
      }
      n479 = Format Into String(format string="Serial=%d\r\n", w987) -> (resulting string=w990:string)  [unwired: 2 in, 1 out]
    }
    frame 52 {
      # "GET_PATIENT_PROGRAM_RUN-TIME"
      n480 = Array To Cluster(array=w1010) -> (cluster=w1011:T6)
      n481 = Unbundle By Name(w1011) -> ("DATA[0]"=w1009:u8, "DATA[5]"=w1006:u8, "DATA[4]"=w1005:u8, "DATA[3]"=w1004:u8, "DATA[2]"=w1003:u8)
      n482 = Join Numbers(hi=w1006, lo=w1005) -> ((hi.lo)=w1008:u16)
      n483 = Join Numbers(hi=w1004, lo=w1003) -> ((hi.lo)=w1007:u16)
      n484 = Join Numbers(hi=w1008, lo=w1007) -> ((hi.lo)=w1002:u32)
      n485 = Format Into String(format string="patientProgramNumber=%d\r\npatientProgramRunTime=%d\r\n", w1009, w1002) -> (resulting string=w1012:string)  [unwired: 2 in, 1 out]
    }
    frame 53 {
      # "SET_PATIENT_PROGRAM_RUN-TIME"
    }
    frame 54 {
      # "IMPEDANCE_MEASUREMENT"
      n486 = Array To Cluster(array=w1018) -> (cluster=w1021:T6)
      n487 = Unbundle By Name(w1021) -> ("DATA[0]"=w1020:u8, "DATA[1]"=w1019:u8, "DATA[3]"=w1017:u8, "DATA[2]"=w1016:u8)
      n488 = Join Numbers(hi=w1017, lo=w1016) -> ((hi.lo)=w1015:u16)
      n489 = Format Into String(format string="channel_A=%d\r\nchannel_B=%d\r\nimpedanceReading=%d\r\n", w1020, w1019, w1015) -> (resulting string=w1022:string)  [unwired: 2 in, 1 out]
    }
    frame 55 {
      # "ENTER_STORAGE_MODE"
    }
    frame 56 {
      # "Echo Short"
      n490 = Array Subset(array=w1028, index=0, length=8) -> (w1026:u8[])
      n491 = Byte Array To String(unsigned byte array=w1026) -> (string=w1025:string)
      n492 = Format Into String(format string="%s", w1025) -> (resulting string=w1030:string)  [unwired: 2 in, 1 out]
    }
    frame 57 {
      # "Echo Long"
      n493 = Array Subset(array=w1033, index=0, length=256) -> (w1034:u8[])
      n494 = Byte Array To String(unsigned byte array=w1034) -> (string=w1032:string)
      n495 = Format Into String(format string="%s", w1032) -> (resulting string=w1037:string)  [unwired: 2 in, 1 out]
    }
    frame 58 {
      # "GET_GENERAL_CALIBRATION"
      n496 = Array Subset(array=w1054, index=0, length=30) -> (w1083:u8[])
      n497 = Array Subset(array=w1054, index=30, length=24) -> (w1053:u8[])
      n498 = Array Subset(array=w1054, index=54, length=30) -> (w1078:u8[])
      n499 = Array Subset(array=w1054, index=80, length=18) -> (w1075:u8[])
      n500 = Array Subset(array=w1054, index=92, length=18) -> (w1073:u8[])
      n501 = Index Array(array=w1054, index=109) -> (element=w1065:u8)
      n502 = Index Array(array=w1054, index=108) -> (element=w1066:u8)
      n503 = call "Process Data In 2 Byte Chunks.vi"("DATA IN"=w1053) -> ("Data Out"=w1051:u16[])  [unwired: 10 in]
      n504 = Join Numbers(hi=w1065, lo=w1066) -> ((hi.lo)=w1064:u16)
      n505 = Index Array(array=w1051) -> (element #1=w1050:u16, element #2=w1049:u16, element #3=w1048:u16, element #4=w1047:u16, element #5=w1046:u16, element #6=w1045:u16, element #7=w1044:u16, element #8=w1043:u16, element #9=w1042:u16, element #10=w1041:u16, element #11=w1040:u16, element #12=w1039:u16)  [unwired: 12 in]
      n506 = for {
        N: 15 -> [_]
        shift-right: [w1141] -> w1081
        shift-left: "" -> [w1142]
        tunnel: w1083 -> [w1139]
        i -> [w1137]
        w1129 = 2 ("index")
        n507 = Multiply(x=w1137, y=w1129) -> (x*y=w1138:i32)
        n508 = Add(x=w1138, y=4) -> (x+y=w1136:i32)
        n509 = Array Subset(array=w1139, index=w1136, length=w1129) -> (w1135:u8[])
        n510 = Array To Cluster(array=w1135) -> (cluster=w1132:cluster{"[0]":u8, "[1]":u8})
        n511 = Unbundle By Name(w1132) -> ("[1]"=w1130:u8, "[0]"=w1131:u8)
        n512 = Join Numbers(hi=w1130, lo=w1131) -> ((hi.lo)=w1133:u16)
        n513 = Format Into String(format string="Reserved[%02d]=0x%02x\r\n", initial string=w1142, w1137, w1133) -> (resulting string=w1141:string)  [unwired: 1 in, 1 out]
      }
      n514 = for {
        N: 15 -> [_]
        shift-right: [w1127] -> w1077
        shift-left: "" -> [w1128]
        tunnel: w1078 -> [w1125]
        i -> [w1123]
        w1115 = 2 ("index")
        n515 = Multiply(x=w1123, y=w1115) -> (x*y=w1124:i32)
        n516 = Add(x=w1124, y=4) -> (x+y=w1122:i32)
        n517 = Array Subset(array=w1125, index=w1122, length=w1115) -> (w1121:u8[])
        n518 = Array To Cluster(array=w1121) -> (cluster=w1118:cluster{"[0]":u8, "[1]":u8})
        n519 = Unbundle By Name(w1118) -> ("[1]"=w1116:u8, "[0]"=w1117:u8)
        n520 = Join Numbers(hi=w1116, lo=w1117) -> ((hi.lo)=w1119:u16)
        n521 = Format Into String(format string="Reserved[%02d]=0x%02x\r\n", initial string=w1128, w1123, w1119) -> (resulting string=w1127:string)  [unwired: 1 in, 1 out]
      }
      n522 = for {
        N: 6 -> [_]
        shift-right: [w1113] -> w1070
        shift-left: "" -> [w1114]
        tunnel: w1075 -> [w1111]
        i -> [w1109]
        w1101 = 2 ("index")
        n523 = Multiply(x=w1109, y=w1101) -> (x*y=w1110:i32)
        n524 = Add(x=w1110, y=4) -> (x+y=w1108:i32)
        n525 = Array Subset(array=w1111, index=w1108, length=w1101) -> (w1107:u8[])
        n526 = Array To Cluster(array=w1107) -> (cluster=w1104:cluster{"[0]":u8, "[1]":u8})
        n527 = Unbundle By Name(w1104) -> ("[1]"=w1102:u8, "[0]"=w1103:u8)
        n528 = Join Numbers(hi=w1102, lo=w1103) -> ((hi.lo)=w1105:u16)
        n529 = Format Into String(format string="batteryStateCalStimOff[%02d]=0x%02x\r\n", initial string=w1114, w1109, w1105) -> (resulting string=w1113:string)  [unwired: 1 in, 1 out]
      }
      n530 = for {
        N: 6 -> [_]
        shift-right: [w1099] -> w1069
        shift-left: "" -> [w1100]
        tunnel: w1073 -> [w1097]
        i -> [w1095]
        w1087 = 2 ("index")
        n531 = Multiply(x=w1095, y=w1087) -> (x*y=w1096:i32)
        n532 = Add(x=w1096, y=4) -> (x+y=w1094:i32)
        n533 = Array Subset(array=w1097, index=w1094, length=w1087) -> (w1093:u8[])
        n534 = Array To Cluster(array=w1093) -> (cluster=w1090:cluster{"[0]":u8, "[1]":u8})
        n535 = Unbundle By Name(w1090) -> ("[1]"=w1088:u8, "[0]"=w1089:u8)
        n536 = Join Numbers(hi=w1088, lo=w1089) -> ((hi.lo)=w1091:u16)
        n537 = Format Into String(format string="batteryStateCalStimOn[%02d]=0x%02x\r\n", initial string=w1100, w1095, w1091) -> (resulting string=w1099:string)  [unwired: 1 in, 1 out]
      }
      n538 = Format Into String(format string="%stempMinThreshold=0x%02x\r\ntempWarningThresholdl=0x%02x\r\ntempCriticalThresholdl=0x%02x\r\ntempAbortThresholdl=0x%02x\r\nthermOffsetMinimum=0x%02x\r\nthermOffsetMaximum=0x%02x\r\nthermBiasMinimum=0x%02x\r\nthermBiasMaximum=0x%02x\r\nthermInputMinimum=0x%02x\r\nthermInputMaximum=0x%02x\r\nbatteryIncreasePreCharge=0x%02x\r\nbatteryIncreaseConstandCurrent=0x%02x\r\n%s%s%svrectMeasurementCal=0x%02x\r\n", w1081, w1050, w1049, w1048, w1047, w1046, w1045, w1044, w1043, w1042, w1041, w1040, w1039, w1077, w1070, w1069, w1064) -> (resulting string=w1085:string)  [unwired: 2 in, 1 out]
    }
    frame 59 {
      # "SET_GENERAL_CALIBRATION"
    }
    frame 60 {
      # "GET_TRIM_LIST"
      n539 = Array To Cluster(array=w1144) -> (cluster=w1149:T6)
      n540 = Unbundle By Name(w1149) -> ("DATA[0]"=w1147:u8, "DATA[1]"=w1146:u8)
      n541 = case shown="0, Default" w1147 {
        tunnel: w1144 -> [w1154 w1179]
        tunnel: [w1152 w1177] -> w1148
        tunnel: w1146 -> [w1151 _]
        frame 0, Default {
          n542 = for {
            N: w1151 -> [_]
            shift-right: [w1168] -> w1152
            shift-left: "" -> [w1169]
            tunnel: w1154 -> [w1166]
            i -> [w1164]
            w1157 = 3 ("index")
            n543 = Multiply(x=w1164, y=w1157) -> (x*y=w1165:i32)
            n544 = Add(x=w1165, y=2) -> (x+y=w1163:i32)
            n545 = Array Subset(array=w1166, index=w1163, length=w1157) -> (w1162:u8[])
            n546 = Array To Cluster(array=w1162) -> (cluster=w1160:cluster{"[0]":u8, "[1]":u8, "[2]":u8})
            n547 = Unbundle By Name(w1160) -> ("[1]"=w1158:u8, "[0]"=w1159:u8, "[2]"=w1155:u8)
            n548 = Join Numbers(hi=w1158, lo=w1159) -> ((hi.lo)=w1156:u16)
            n549 = Format Into String(format string="Address=0x%04x\r\nData=0x%02x\r\n", initial string=w1169, w1156, w1155) -> (resulting string=w1168:string)  [unwired: 1 in, 1 out]
          }
        }
        frame 2 {
          n550 = Array To Cluster(array=w1179) -> (cluster=w1180:T12)
          n551 = Unbundle By Name(w1180) -> ("DATA[2]"=w1178:u8, "DATA[3]"=w1176:u8, "DATA[4]"=w1175:u8, "DATA[5]"=w1174:u8, "DATA[6]"=w1173:u8, "DATA[7]"=w1172:u8, "DATA[8]"=w1171:u8)
          n552 = Join Numbers(hi=w1172, lo=w1171) -> ((hi.lo)=w1170:u16)
          n553 = Format Into String(format string="BG_TRIM=0x%02x\r\nPGO_TRIM=0x%02x\r\nCASN_TRIM=0x%02x\r\nCASP_TRIM=0x%02x\r\nHVDDL_TRIM=0x%02x\r\nGLOBAL_GAIN_TRIM=0x%04x\r\n", w1178, w1176, w1175, w1174, w1173, w1170) -> (resulting string=w1177:string)  [unwired: 2 in, 1 out]
        }
      }
      n554 = Format Into String(format string="ListNum=%d\r\nListLen=%d\r\n%s", w1147, w1146, w1148) -> (resulting string=w1145:string)  [unwired: 2 in, 1 out]
    }
    frame 61 {
      # "SET_TRIM_LIST"
    }
    frame 62 {
      # "GET_COUNTER"
      n555 = Array To Cluster(array=w1192) -> (cluster=w1191:T4)
      n556 = Unbundle By Name(w1191) -> ("DATA[0]"=w1190:u8, "DATA[2]"=w1188:u8, "DATA[3]"=w1189:u8, "DATA[4]"=w1186:u8, "DATA[5]"=w1187:u8)
      n557 = Join Numbers(hi=w1187, lo=w1186) -> ((hi.lo)=w1185:u16)
      n558 = Join Numbers(hi=w1189, lo=w1188) -> ((hi.lo)=w1184:u16)
      n559 = Join Numbers(hi=w1185, lo=w1184) -> ((hi.lo)=w1183:u32)
      n560 = Format Into String(format string="eventCounterID=%d\r\neventCount=%d\r\n", w1190, w1183) -> (resulting string=w1193:string)  [unwired: 2 in, 1 out]
    }
    frame 63 {
      # "SET_COUNTER"
    }
    frame 64 {
      # "GET_TEST_STIMULATION"
      n561 = Index Array(array=w1197, index #1=0 ("index")) -> (element #1=w1200:u8, element #2=w1199:u8, element #3=w1198:u8)  [unwired: 2 in]
      n562 = for {
        N: 4 -> [_]
        shift-right: [w1237] -> w1196
        shift-left: "" -> [w1238]
        tunnel: w1197 -> [w1227]
        i -> [w1228]
        w1207 = 8 ("index")
        w1242 = 35 ("length")
        n563 = Multiply(x=w1228, y=w1242) -> (x*y=w1240:i32)
        n564 = Add(x=3 ("index"), y=w1240) -> (x+y=w1241:i32)
        n565 = Array Subset(array=w1227, index=w1241, length=w1242) -> (w1225:u8[])
        n566 = Array To Cluster(array=w1225) -> (cluster=w1220:T13)
        n567 = Array Subset(array=w1225, index=5, length=26) -> (w1231:u8[])
        n568 = Unbundle By Name(w1220) -> ("[31]"=w1219:u8, "[32]"=w1218:u8, "[33]"=w1217:u8, "[34]"=w1214:u8, "[35]"=w1213:u8, "[36]"=w1209:u8, "[37]"=w1208:u8)
        n569 = Unbundle By Name(w1220) -> ("[3]"=w1223:u8, "[4]"=w1224:u8)
        n570 = To Unsigned Word Integer(number=w1224) -> (unsigned 16bit integer=w1236:u16)
        n571 = for {
          N: 26 -> [_]
          tunnel: w1231 -> [w1243] mode=indexing
          shift-right: [w1249] -> w1221
          shift-left: "" -> [w1250]
          tunnel: w1228 -> [w1244]
          i -> [w1247]
          n572 = case shown="3" w1244 {
            tunnel: ["ChannelPercentagePA[CH%02d]=%d\\r\\n" ("format string") "ChannelPercentagePB[CH%02d]=%d\\r\\n" ("format string") "ChannelPercentagePC[CH%02d]=%d\\r\\n" ("format string") "ChannelPercentagePD[CH%02d]=%d\\r\\n" ("format string")] -> w1248
            frame 0, Default {
            }
            frame 1 {
            }
            frame 2 {
            }
            frame 3 {
            }
          }
          n573 = To Byte Integer(number=w1243) -> (8bit integer=w1245:i8)
          n574 = Increment(x=w1247) -> (x+1=w1246:i32)
          n575 = Format Into String(format string=w1248, initial string=w1250, w1246, w1245) -> (resulting string=w1249:string)  [unwired: 1 in, 1 out]
        }
        n576 = To Unsigned Word Integer(number=w1213) -> (unsigned 16bit integer=w1215:u16)
        n577 = To Unsigned Word Integer(number=w1208) -> (unsigned 16bit integer=w1211:u16)
        n578 = Logical Shift(y=8 ("index"), x=w1236) -> (x << y=w1235:u16)
        n579 = Logical Shift(y=w1207, x=w1215) -> (x << y=w1216:u16)
        n580 = Logical Shift(y=w1207, x=w1211) -> (x << y=w1210:u16)
        n581 = Add(x=w1223, y=w1235) -> (x+y=w1222:u16)
        n582 = Add(x=w1214, y=w1216) -> (x+y=w1212:u16)
        n583 = Add(x=w1209, y=w1210) -> (x+y=w1206:u16)
        n584 = Format Into String(format string="\r\n-- PULSE PB --\r\nAmplitude=%d\r\n%s\r\nStimWidth=%d\r\nInterphaseDelay=%d\r\nRecoveryRatioSelect=%d\r\nPassiveRecoveryWidth=%d\r\nCBCWidth=%d", initial string=w1238, w1222, w1221, w1219, w1218, w1217, w1212, w1206) -> (resulting string=w1237:string)  [unwired: 1 in, 1 out]
      }
      n585 = Format Into String(format string="FrequencyIndex=%d\r\nComplianceVoltage=%d\r\nNumPulses=%d\r\n%s", w1200, w1199, w1198, w1196) -> (resulting string=w1205:string)  [unwired: 2 in, 1 out]
    }
    frame 65 {
      # "SET_TEST_STIMULATION"
    }
    frame 66 {
      # "GET_TITRATION_STIMULATION"
      n586 = Index Array(array=w1257, index #1=0 ("index")) -> (element #1=w1261:u8, element #2=w1260:u8)  [unwired: 1 in]
      n587 = for {
        N: 4 -> [_]
        shift-right: [w1287] -> w1256
        shift-left: "" -> [w1288]
        tunnel: w1257 -> [w1278]
        i -> [w1279]
        w1267 = 8 ("index")
        w1292 = 30 ("length")
        n588 = Multiply(x=w1279, y=w1292) -> (x*y=w1290:i32)
        n589 = Add(x=2 ("index"), y=w1290) -> (x+y=w1291:i32)
        n590 = Array Subset(array=w1278, index=w1291, length=w1292) -> (w1276:u8[])
        n591 = Array To Cluster(array=w1276) -> (cluster=w1272:T14)
        n592 = Array Subset(array=w1276, index=6, length=26) -> (w1282:u8[])
        n593 = Unbundle By Name(w1272) -> ("[2]"=w1274:u8, "[3]"=w1275:u8, "[4]"=w1269:u8, "[5]"=w1268:u8)
        n594 = To Unsigned Word Integer(number=w1275) -> (unsigned 16bit integer=w1286:u16)
        n595 = To Unsigned Word Integer(number=w1268) -> (unsigned 16bit integer=w1270:u16)
        n596 = for {
          N: 26 -> [_]
          tunnel: w1282 -> [w1293] mode=indexing
          shift-right: [w1299] -> w1265
          shift-left: "" -> [w1300]
          tunnel: w1279 -> [w1294]
          i -> [w1297]
          n597 = case shown="3" w1294 {
            tunnel: ["channelPercentagePA[CH%02d]=%d\\r\\n" ("format string") "channelPercentagePB[CH%02d]=%d\\r\\n" ("format string") "channelPercentagePC[CH%02d]=%d\\r\\n" ("format string") "channelPercentagePD[CH%02d]=%d\\r\\n" ("format string")] -> w1298
            frame 0, Default {
            }
            frame 1 {
            }
            frame 2 {
            }
            frame 3 {
            }
          }
          n598 = To Byte Integer(number=w1293) -> (8bit integer=w1295:i8)
          n599 = Increment(x=w1297) -> (x+1=w1296:i32)
          n600 = Format Into String(format string=w1298, initial string=w1300, w1296, w1295) -> (resulting string=w1299:string)  [unwired: 1 in, 1 out]
        }
        n601 = Logical Shift(y=w1267, x=w1286) -> (x << y=w1285:u16)
        n602 = Logical Shift(y=w1267, x=w1270) -> (x << y=w1271:u16)
        n603 = Add(x=w1274, y=w1285) -> (x+y=w1273:u16)
        n604 = Add(x=w1269, y=w1271) -> (x+y=w1266:u16)
        n605 = Format Into String(format string="\r\n-- TITR_PULSE PB --\r\nAmplitude=%d\r\npulseWidth=%d\r\n%s", initial string=w1288, w1273, w1266, w1265) -> (resulting string=w1287:string)  [unwired: 1 in, 1 out]
      }
      n606 = Format Into String(format string="frequencyIndex=%d\r\nnumPulses=%d\r\n%s", w1261, w1260, w1256) -> (resulting string=w1264:string)  [unwired: 2 in, 1 out]
    }
    frame 67 {
      # "SET_TITRATION_STIMULATION"
    }
    frame 68 {
      # "GET_RAMP_TIME"
      n607 = Array To Cluster(array=w1313) -> (cluster=w1312:cluster{"DATA[0]":u8, "DATA[1]":u8})
      n608 = Unbundle By Name(w1312) -> ("DATA[0]"=w1309:u8, "DATA[1]"=w1308:u8)
      n609 = To Unsigned Word Integer(number=w1308) -> (unsigned 16bit integer=w1307:u16)
      n610 = Logical Shift(y=8 ("index"), x=w1307) -> (x << y=w1311:u16)
      n611 = Add(x=w1309, y=w1311) -> (x+y=w1306:u16)
      n612 = Format Into String(format string="RampTime=%d\r\n", w1306) -> (resulting string=w1314:string)  [unwired: 2 in, 1 out]
    }
    frame 69 {
      # "SET_RAMP_TIME"
    }
    frame 70 {
      # "GET_VBAT"
      n613 = Array To Cluster(array=w1318) -> (cluster=w1324:cluster{"DATA[0]":u8, "DATA[1]":u8})
      n614 = Unbundle By Name(w1324) -> ("DATA[0]"=w1321:u8, "DATA[1]"=w1320:u8)
      n615 = To Unsigned Word Integer(number=w1320) -> (unsigned 16bit integer=w1319:u16)
      n616 = Logical Shift(y=8 ("index"), x=w1319) -> (x << y=w1323:u16)
      n617 = Add(x=w1321, y=w1323) -> (x+y=w1317:u16)
      n618 = Format Into String(format string="vbat=%d\r\n", w1317) -> (resulting string=w1326:string)  [unwired: 2 in, 1 out]
    }
    frame 71 {
      # "Not yet documented"
      # "SET_SOFTWARE_DESCRIPTION_BLOCK"
    }
    frame 72 {
      # "Not yet documented"
      # "GET_SOFTWARE_DESCRIPTION_BLOCK"
    }
    frame 73 {
      # "WRITE_MEMORY"
    }
    frame 74 {
      # "READ_MEMORY"
      n619 = Array To Cluster(array=w1336) -> (cluster=w1352:T15)
      n620 = Unbundle By Name(w1352) -> ("DATA[3]"=w1349:u8, "DATA[2]"=w1348:u8, "DATA[1]"=w1347:u8, "DATA[0]"=w1346:u8, "DATA[4]"=w1338:u8, "DATA[5]"=w1339:u8)
      n621 = Array Subset(array=w1336, index=6, length=64 ("index")) -> (w1333:u8[])
      n622 = Join Numbers(hi=w1349, lo=w1348) -> ((hi.lo)=w1351:u16)
      n623 = Join Numbers(hi=w1347, lo=w1346) -> ((hi.lo)=w1350:u16)
      n624 = Byte Array To String(unsigned byte array=w1333) -> (string=w1330:string)
      n625 = To Unsigned Word Integer(number=w1339) -> (unsigned 16bit integer=w1340:u16)
      n626 = Index Array(array=w1333, index #1=0 ("index"), index #2=1 ("index")) -> (element #1=w1331:u8, element #2=w1328:u8)
      n627 = Join Numbers(hi=w1351, lo=w1350) -> ((hi.lo)=w1343:u32)
      n628 = Logical Shift(y=8 ("index"), x=w1340) -> (x << y=w1342:u16)
      n629 = Add(x=w1338, y=w1342) -> (x+y=w1337:u16)
      n630 = Format Into String(format string="address=%d\r\nlength=%d\r\ndata0=%d\r\ndata1=%d\r\n%s", w1343, w1337, w1331, w1328, w1330) -> (resulting string=w1344:string)  [unwired: 2 in, 1 out]
    }
    frame 75 {
      # "Not yet documented"
      # "RESET_xPG"
    }
    frame 76 {
      # "Not yet documented"
      # "ERASE_FLASH_BLOCK"
    }
    frame 77 {
      # "Not yet documented"
      # "WRITE_VECTORS"
    }
    frame 78 {
      # "Not yet documented"
      # "READ_VECTORS"
    }
    frame 79 {
      # "DIAGNOSTIC_DATA"
      n631 = Index Array(array=w1353, index=1) -> (element=w1355:u8)
      n632 = case shown="2" w1355 {
        tunnel: [w1367 "Unsupported State" w1384 w1401] -> w1354
        tunnel: w1353 -> [w1364 _ w1383 w1393]
        frame 0, 1 {
          # "Capacitor Data, BG Impedance"
          n633 = Array Subset(array=w1364, index=2, length=53) -> (w1362:u8[])
          n634 = for {
            N: 26 -> [_]
            shift-right: [w1379] -> w1360
            shift-left: w1362 -> [w1381]
            shift-right: [w1368] -> w1357
            shift-left: "" -> [w1369]
            i -> [w1372]
            n635 = Split 1D Array(array=w1381, index=2) -> (first subarray=w1378:u8[], second subarray=w1379:u8[])
            n636 = Increment(x=w1372) -> (x+1=w1371:i32)
            n637 = Index Array(array=w1378, index #1=1 ("index"), index #2=0 ("index")) -> (element #1=w1374:u8, element #2=w1375:u8)
            n638 = Join Numbers(hi=w1374, lo=w1375) -> ((hi.lo)=w1370:u16)
            n639 = Format Into String(format string="Channel%d Voltage=%d\\r\\n", initial string=w1369, w1371, w1370) -> (resulting string=w1368:string)  [unwired: 1 in, 1 out]
          }
          n640 = Index Array(array=w1360) -> (element=w1358:u8)  [unwired: 1 in]
          n641 = Format Into String(format string="%sData Valid=%d", w1357, w1358) -> (resulting string=w1367:string)  [unwired: 2 in, 1 out]
        }
        frame 5, Default {
        }
        frame 2 {
          # "VBat Data"
          n642 = Array To Cluster(array=w1383) -> (cluster=w1386:T6)
          n643 = Unbundle By Name(w1386) -> ("DATA[3]"=w1387:u8, "DATA[2]"=w1388:u8)
          n644 = Join Numbers(hi=w1387, lo=w1388) -> ((hi.lo)=w1385:u16)
          n645 = Format Into String(format string="VoltageReading=%d\r\n", w1385) -> (resulting string=w1384:string)  [unwired: 2 in, 1 out]
        }
        frame 3 {
          # "Thermistor Data"
          n646 = Array To Cluster(array=w1393) -> (cluster=w1394:T6)
          n647 = Unbundle By Name(w1394) -> ("DATA[3]"=w1399:u8, "DATA[2]"=w1400:u8, "DATA[5]"=w1397:u8, "DATA[4]"=w1398:u8, "DATA[7]"=w1395:u8, "DATA[6]"=w1396:u8)
          n648 = Join Numbers(hi=w1399, lo=w1400) -> ((hi.lo)=w1392:u16)
          n649 = Join Numbers(hi=w1397, lo=w1398) -> ((hi.lo)=w1391:u16)
          n650 = Join Numbers(hi=w1395, lo=w1396) -> ((hi.lo)=w1390:u16)
          n651 = Format Into String(format string="ThermBias=%d\r\nThermInput=%d\r\nThermOffset=%d", w1392, w1391, w1390) -> (resulting string=w1401:string)  [unwired: 2 in, 1 out]
        }
      }
    }
    frame 80 {
      # "SET_BACKGROUND_IMPEDANCE"
    }
    frame 81 {
      # "GET_BACKGROUND_IMPEDANCE"
      n652 = Array To Cluster(array=w1409) -> (cluster=w1408:T16)
      n653 = Unbundle By Name(w1408) -> ("DATA[0]"=w1404:u8, "DATA[1]"=w1406:u8)
      n654 = Greater Than 0?(x=w1406) -> (x > 0?=w1407:bool)
      n655 = case shown="False" w1407 {
        tunnel: ["disabled" "enabled"] -> w1405
        frame False {
        }
        frame True {
        }
      }
      n656 = Format Into String(format string="bgiAmplitude=%d\r\nenabled=%s\r\n", w1404, w1405) -> (resulting string=w1411:string)  [unwired: 2 in, 1 out]
    }
    frame 84 {
      # "TKN_GET_LOG_RANGE"
      n657 = Array To Cluster(array=w1417) -> (cluster=w1428:T4)
      n658 = Array Subset(array=w1417, index=8) -> (w1415:u8[])  [unwired: 1 in]
      n659 = Unbundle By Name(w1428) -> ("DATA[0]"=w1426:u8, "DATA[1]"=w1424:u8, "DATA[2]"=w1425:u8, "DATA[3]"=w1422:u8, "DATA[4]"=w1421:u8, "DATA[5]"=w1420:u8, "DATA[6]"=w1419:u8, "DATA[7]"=w1418:u8)
      n660 = Index Array(array=w1415) -> (element=w1414:u8)  [unwired: 1 in]
      n661 = Format Into String(format string="LogNum=%d\r\nINDEX[1]=%d\r\nINDEX[2]=%d\r\nINDEX[3]=%d\r\nINDEX[4]=%d\r\nINDEX[5]=%d\r\nINDEX[6]=%d\r\nINDEX[7]=%d\r\nmaxSerialNum=%d\r\n", w1426, w1424, w1425, w1422, w1421, w1420, w1419, w1418, w1414) -> (resulting string=w1423:string)  [unwired: 2 in, 1 out]
    }
    frame 92 {
      # "1. Standard response codes.\n2. NO DATA!\n3. RSSI results are placed in the activity log."
      # "TKN_MICS_DIAGNOSTICS"
    }
    frame 32682 {
      # "Undefined"
    }
  }
  n662 = Unbundle By Name(w19) -> ("respToken"=w5:u8, "cmdToken"=w7:u16, "b1ChkSum"=w25:u8, "b1ChkSumCalc"=w24:u8, "tChkSum"=w23:u8, "tChkSumCalc"=w22:u8)
  n663 = call <vilib>:"Trim Whitespace.vi"("string"=w27) -> ("trimmed string"=→"Data":string)  [unwired: 1 in]
  n664 = call "MICS Response Lookup.vi"("Token"=w5) -> ("description"=w3:string, "name"=w4:string)  [unwired: 5 in, 3 out]
  n665 = Equal?(x=w25, y=w24) -> (x = y?=→"bChecksum Valid":bool)
  n666 = Equal?(x=w23, y=w22) -> (x = y?=→"tChecksum Valid":bool)
  n667 = Concatenate Strings(w4, "\n" ("string"), w3) -> (→"Response Code":string)
  n668 = call "MICS Command Lookup.vi"("token"=w7) -> ("command"=→"Response Token":string)  [unwired: 5 in, 4 out]
  "error out" <- "error in (no error)"
